vi "Panorama Generation-samples.vi"() -> ()   [LabVIEW 2023]
uses:
  <vilib>/vision/Image Controls.llb/IMAQ Image.ctl
  <vilib>/vision/Calibration.llb/Distortion Model.ctl
  <vilib>/vision/Calibration.llb/Distortion Model Types.ctl
  <vilib>/vision/EDVR.llb/IMAQ ImageToEDVR 2D SGL.vi
  <vilib>/vision/EDVR.llb/IMAQ ImageToEDVR 2D U8.vi
  <vilib>/vision/NI_Vision_Development_Module.lvlib
panel:
  in  "?":T1(tab)
  in  "?":enum32{"Processing Time  Display Tab"}(tab)
  out "SSIM Flat":dbl
  out "SSIM Original":dbl
  out "Correction":dbl
  out "Flat Fielding":dbl
  out "ROI Blending":dbl
  out "Processed FPS":dbl
  in  "Stop":bool
  out "Original Luma?":bool
  out "Left corrected, adjusted, and wrapped image":T2(plugin-control) caption="Thresholded Grid"
  out "Right corrected, adjusted, and wrapped image":T2(plugin-control) caption="Thresholded Grid"
  out "Right Sample":T2(plugin-control) caption="Thresholded Grid"
  out "Left Sample":T2(plugin-control) caption="Thresholded Grid"
  out "Panorama Image":T2(plugin-control)
  in  "?":enum32{"Tunning Control Tab"}(tab)
  in  "Right Image Name":string="right.png"
  in  "Left Image Name":string="left.png"
  in  "Wrapping Factor":i32=5
  in  "Correction Interpolation":u32(ring) items=["Zero Order", "Bi-Linear", "Quadratic", "Cubic Spline"]
  in  "Grid Path":path
  in  "Blending Method":enum16{"WA", "MBB", "WE"}(ring)
  in  "Grid Name":string="grid.png"
  in  "ROI_X":i32=10
  out "Right corrected, adjusted, and wrapped grid":T2(plugin-control) caption="Right  corrected wrapped grid"
  out "Left corrected, adjusted, and wrapped grid":T2(plugin-control) caption="Left corrected  and wrapped grid"
  out "Thresholded and filtered grid":T2(plugin-control) caption="Thresholded Grid"
  out "Grid Image":T2(plugin-control) caption="Circular Dotted Grid"
  out "ROI_L":T2(plugin-control)
  out "ROI_R":T2(plugin-control)
  out "Blended ROI":T2(plugin-control)
  out "Wrapped Y":i32
  out "Grid X":i32
  out "Grid Y":i32
  out "corrected":T2[](array[typedef])
  out "Adjusted":T2[](array[typedef])
  out "RGB Left":T2[](array[typedef])
  out "RGB Right":T2[](array[typedef])
  out "Y0":dbl
  out "X0":dbl
  out "Y1":dbl
  out "X1":dbl
  out "Y2":dbl
  out "X2":dbl
  out "Wrapped X":i32
  out "GP":T2[][](array[typedef])
  out "LP":T2[][](array[typedef])
  out "Masked RGB Right MBB":T2[](array[typedef])
  out "Masked RGB Left MBB":T2[](array[typedef])
  out "Combined Laplace":T2[][](array[typedef])
  out "Start Time":dbl
  out "Correction End Time":dbl
  out "Flat Fielding End Time":dbl
  out "Blending End Time":dbl
  out "Wrapped":T2[](array[typedef])
  out "error out":errorcluster
  out "corrected size":cluster{"X Resolution":i32, "Y Resolution":i32}
  # "This VI meticulously generates panoramic images through a carefully structured process:\n\nLens Distortion Correction: Specifically addressing Barrel Distortion to ensure precise visual accuracy.\nBrightness Variation Compensation: Achieving a seamless transition by compensating variations in brightness.\nROI Blending: Merging carefully determined Regions of Interest (ROIs) using a selected method (Weighted Average - Default, Multi-Band Blending, Wavelet Extraction).\nFinal Panorama Output: Projecting the corrected and blended elements to produce the ultimate panorama.\n\nUser Steps: Navigate to the \"Tuning Control Tab\" and follow these steps:\n\nSelect Grid Image Path: Specify the path for the grid image.\nInput Grid Image Name: Enter the grid image name as saved in the device, including its extension.\nChoose Left and Right Cameras: Indicate the cameras for the left and right images.\nCorrection Interpolation Type: Determine the interpolation type for the correction process (Zero-Order, or Bilinear).\nSet Wrapping Factor: Define the wrapping factor based on the angle between the cameras.\nROI Resolution: Specify the resolution for the Regions of Interest (ROIs).\nBlending Method: Select the preferred blending method (Weighted Average - Default, Multi-Band Blending, Wavelet Extraction).\nRun the VI."
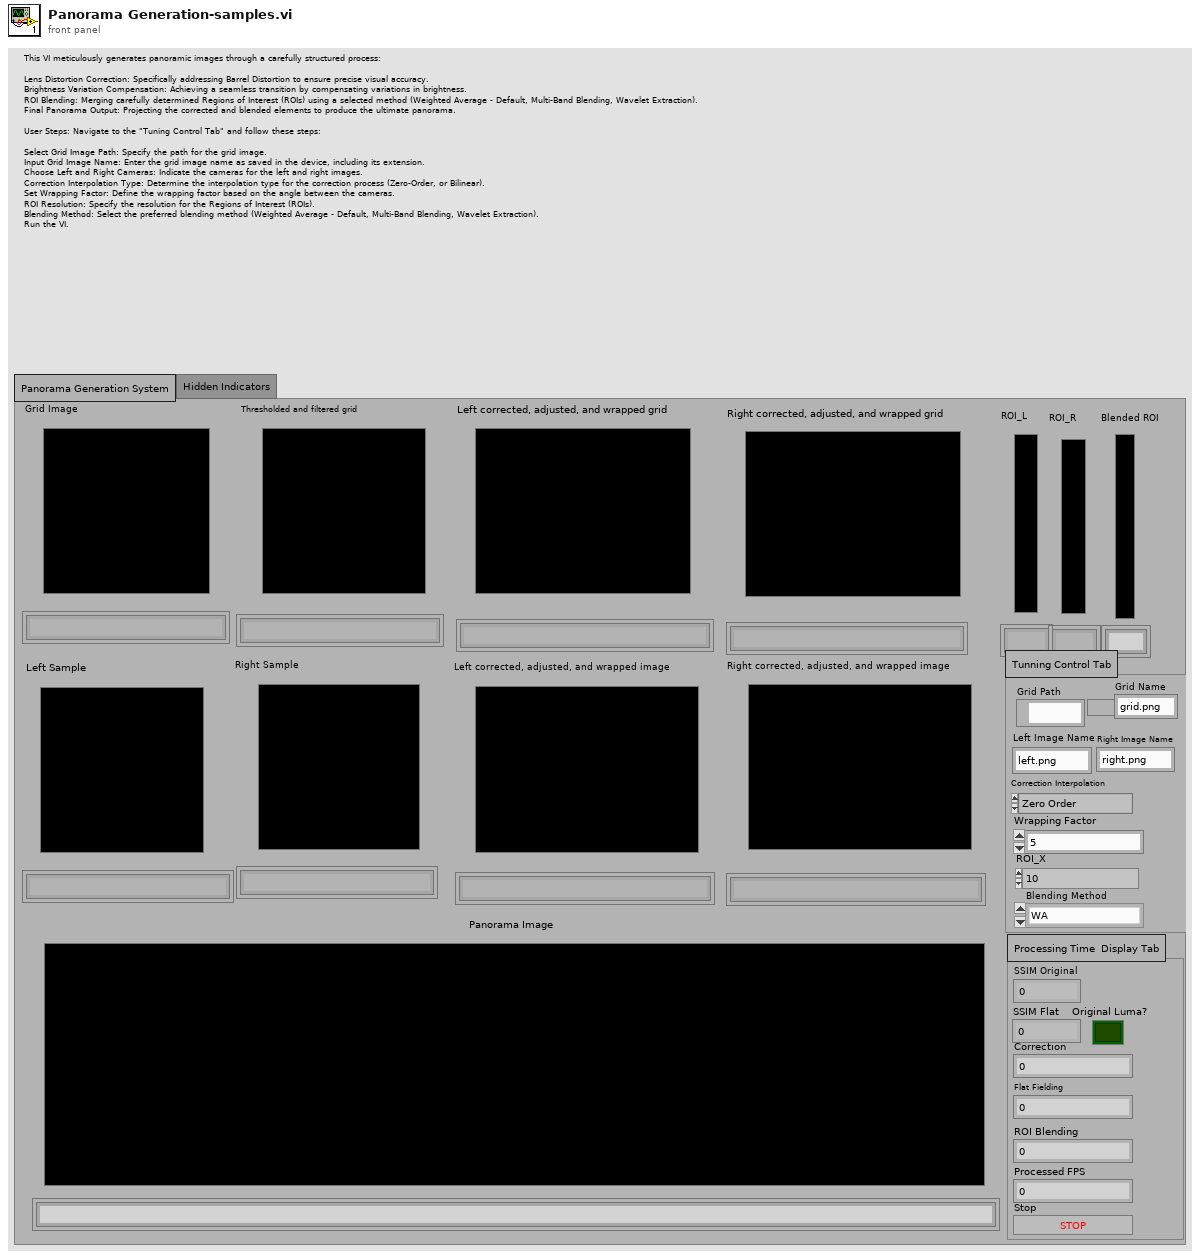
[diagram p1: front panel]
types:
  T1 = enum32{"Panorama Generation System", "Hidden Indicators"}
  T2 = typedef "IMAQ Image.ctl" = refnum<image>
  T3 = typedef "Image Unit" = enum32{"Undefined", "Angström", "Micrometer", "Millimeter", "Centimeter", "Meter", "Kilometer", "Microinch", "Inch", "Feet", "Nautical miles", "Standard miles", "Steps"}
  T4 = typedef "Particle Parameters" = i32
  T5 = cluster{"Measurement Parameter":T4, "Range Lower Value":dbl, "Range Upper Value":dbl, "Range":bool, "Measurement Type":bool}[]
  T6 = cluster{"Corrected Image Scaling":u32, "Corrected Image Learn ROI":u32, "Learn Correction Table?":bool}
  T7 = typedef "Distortion Model.ctl" = cluster{"Distortion Model":T8, "Polynomial Model Setup":cluster{"Radial Coefficient":u32, "Tangential Coefficients ":bool}}
  T8 = typedef "Distortion Model Types.ctl" = i32
  T9 = typedef "Image Type" = u32
  T10 = typedef "Calibration Reference Points.ctl" = cluster{"Pixel Coordinates":cluster{"X":dbl, "Y":dbl}[], "Real World Coordinates":cluster{"X":dbl, "Y":dbl}[], "Unit":T3, "Image Size":cluster{"X":u32, "Y":u32}}
  T11 = cluster{cluster{"element":dbl, "element":dbl}[], cluster{"element":dbl, "element":dbl}[], "Unit":T3, cluster{"X Resolution":i32, "Y Resolution":i32}}
  T12 = cluster{"Model":i32, "corrected size":cluster{"X Resolution":i32, "Y Resolution":i32}, "Polynomial Degree":i32}
  T13 = cluster{"Estimate Background?":bool, "Method":i32, "Polynomial Degree":i32, "corrected size":cluster{"X Resolution":i32, "Y Resolution":i32}, "Niblack Deviation Factor (0.2)":dbl}
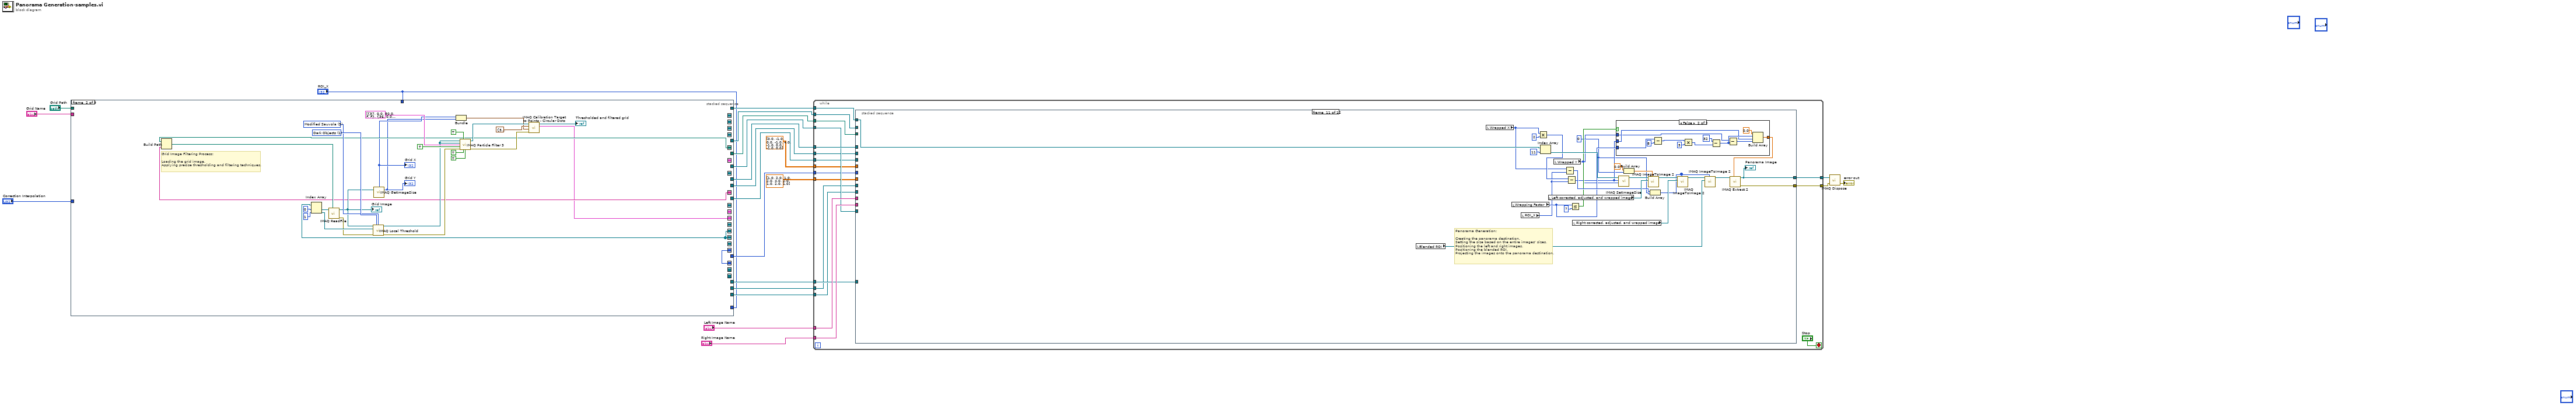
[diagram p0: block diagram]
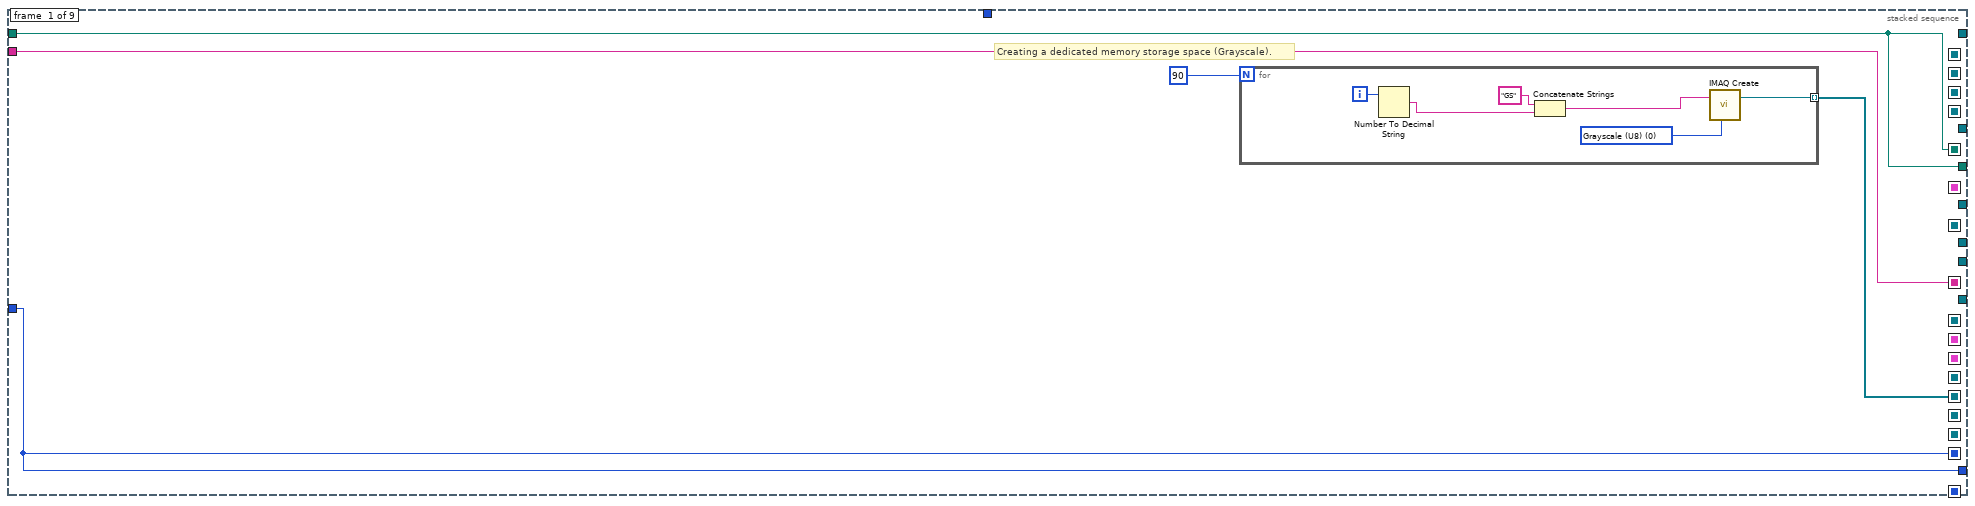
[diagram p2: hidden frame]
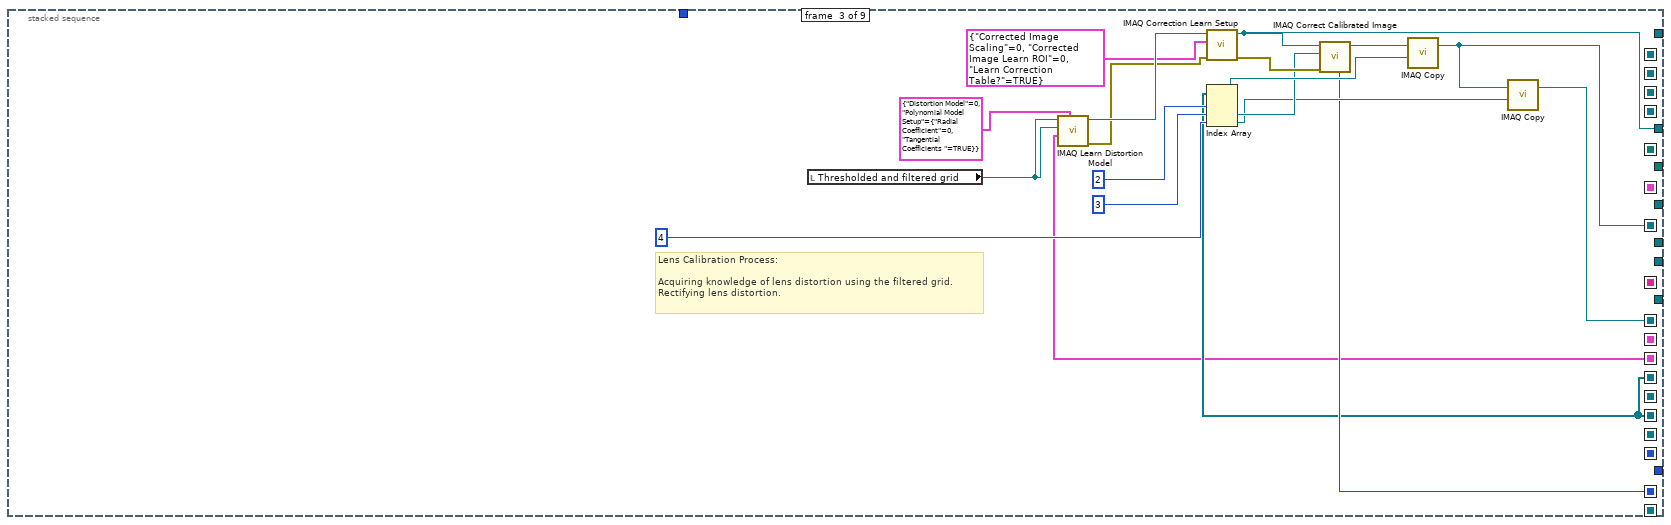
[diagram p3: hidden frame]
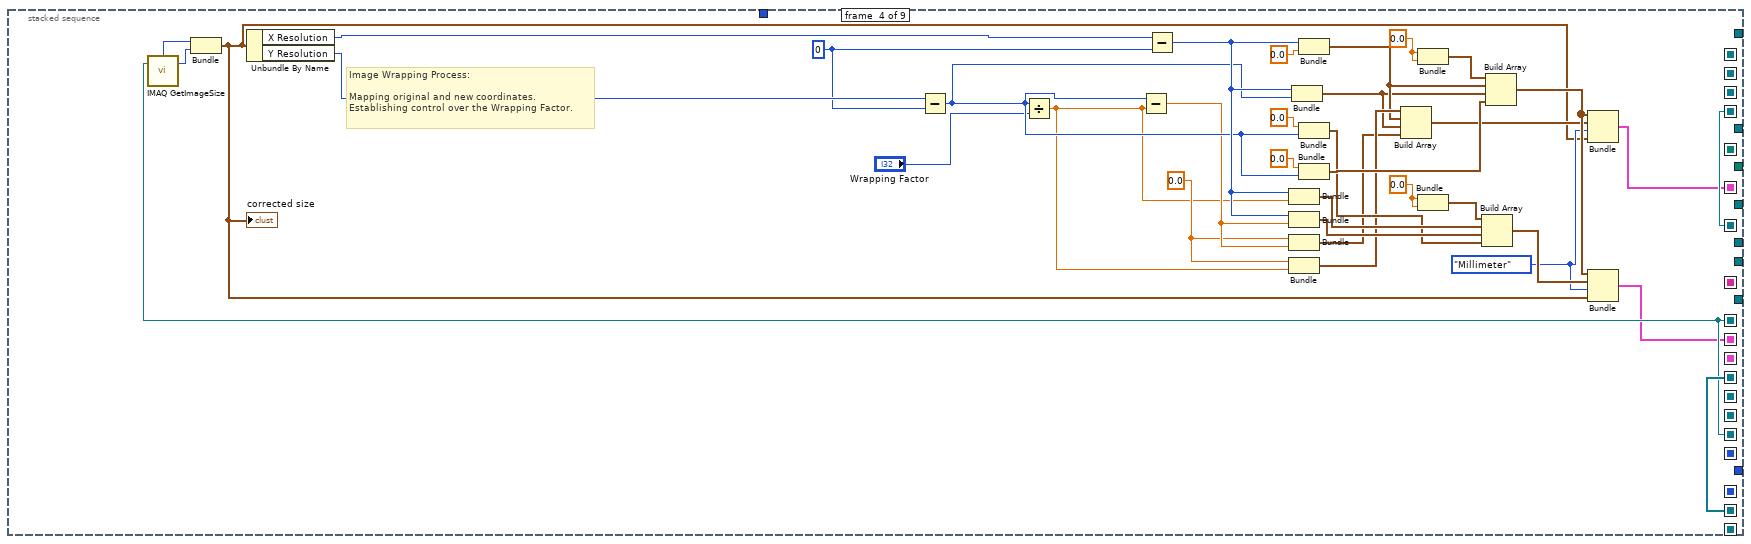
[diagram p4: hidden frame]
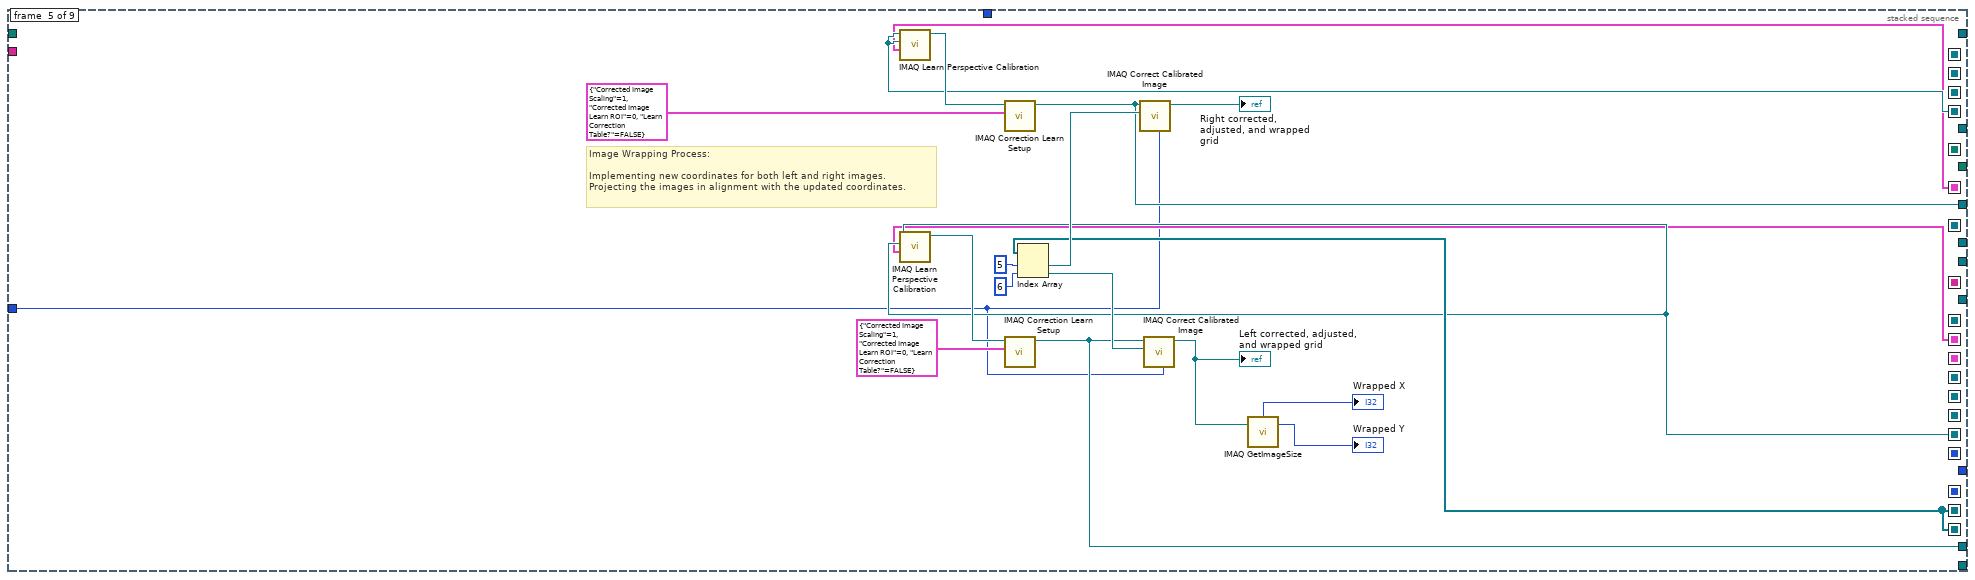
[diagram p5: hidden frame]
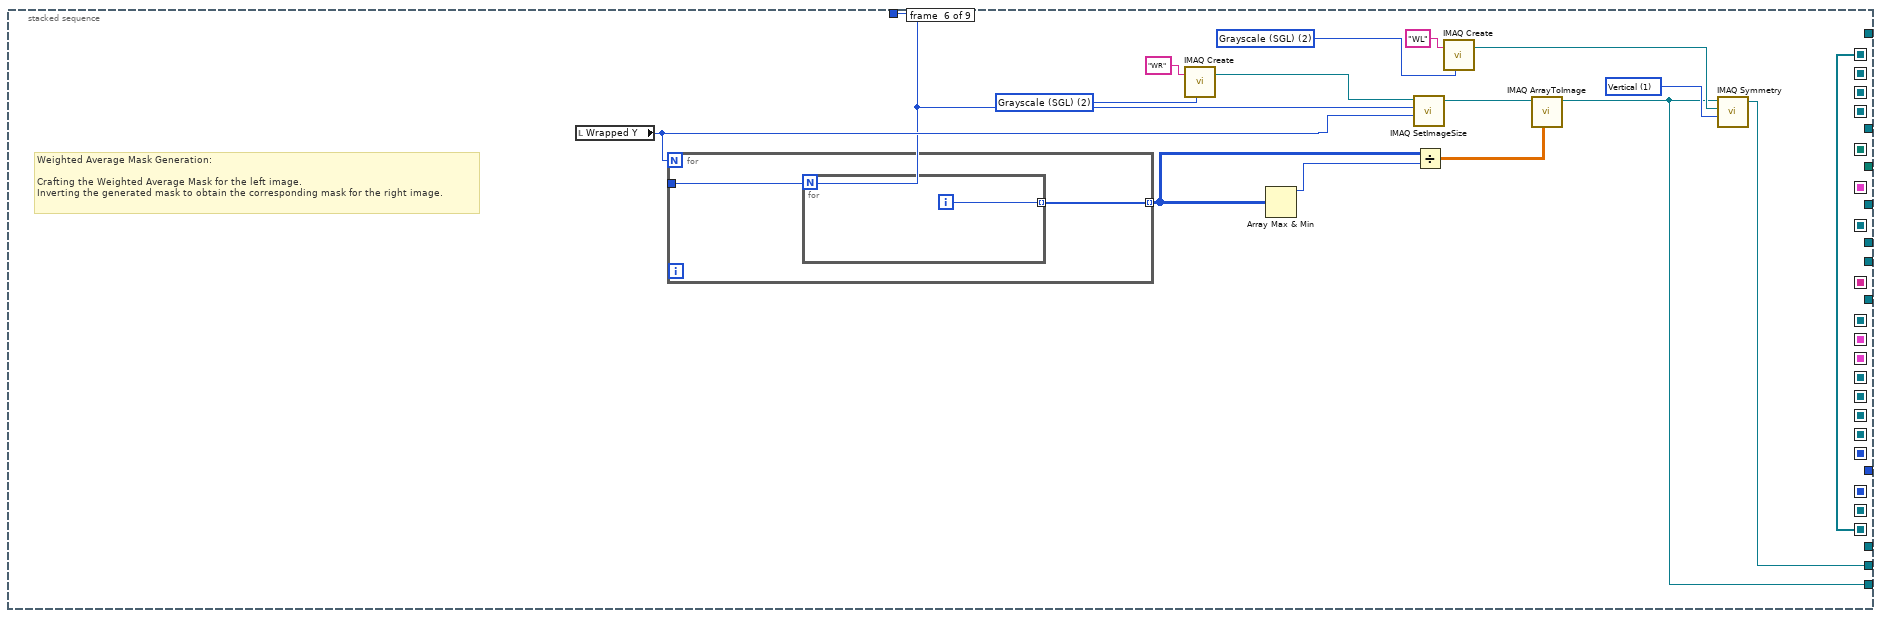
[diagram p6: hidden frame]
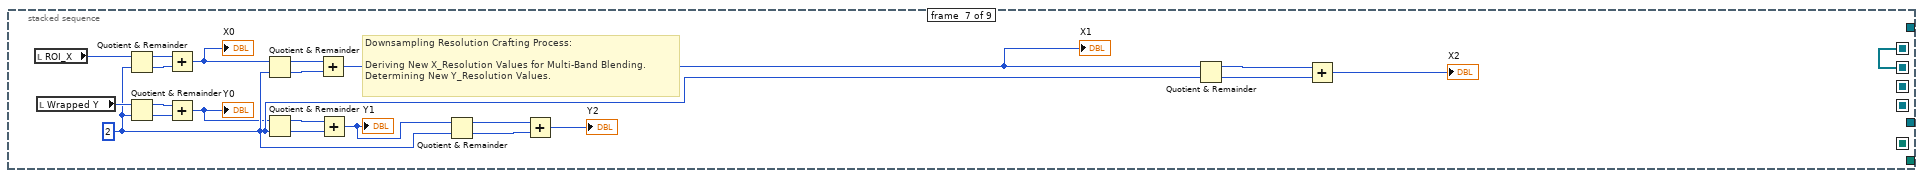
[diagram p7: hidden frame]
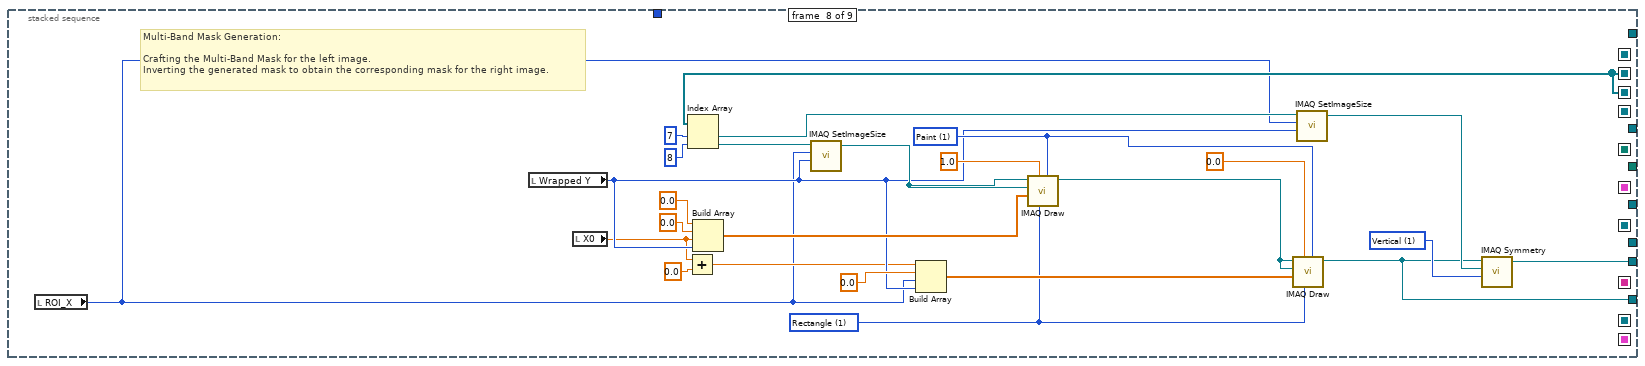
[diagram p8: hidden frame]
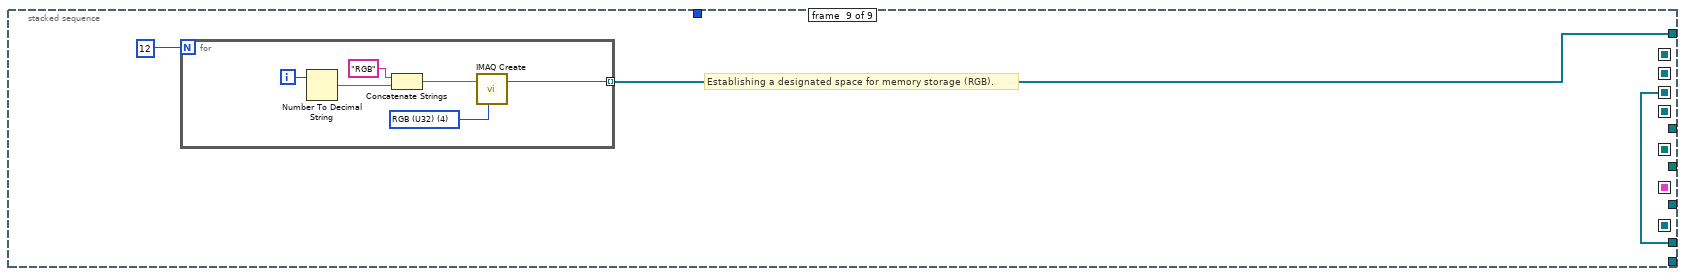
[diagram p9: hidden frame]
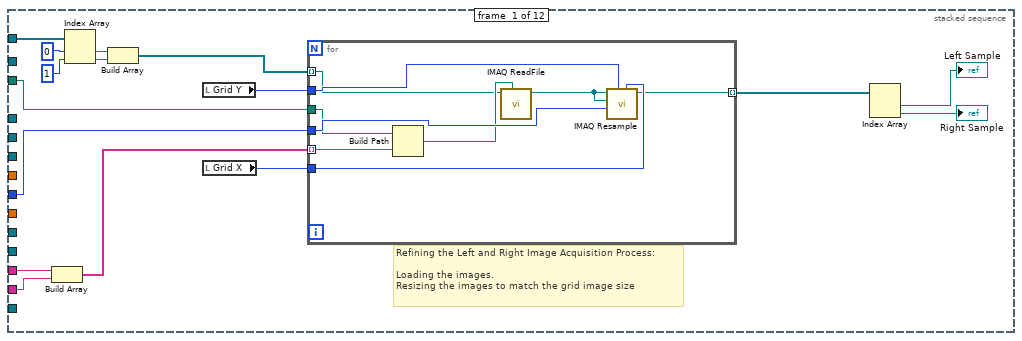
[diagram p10: hidden frame]
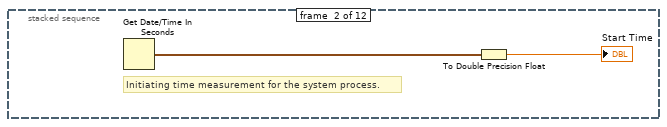
[diagram p11: hidden frame]
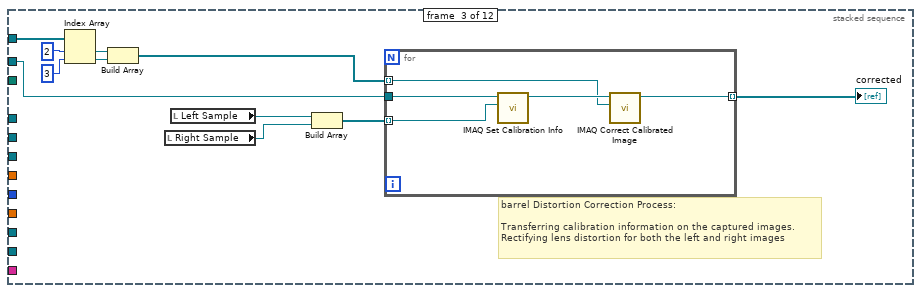
[diagram p12: hidden frame]
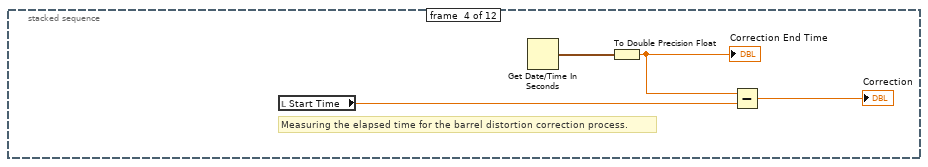
[diagram p13: hidden frame]
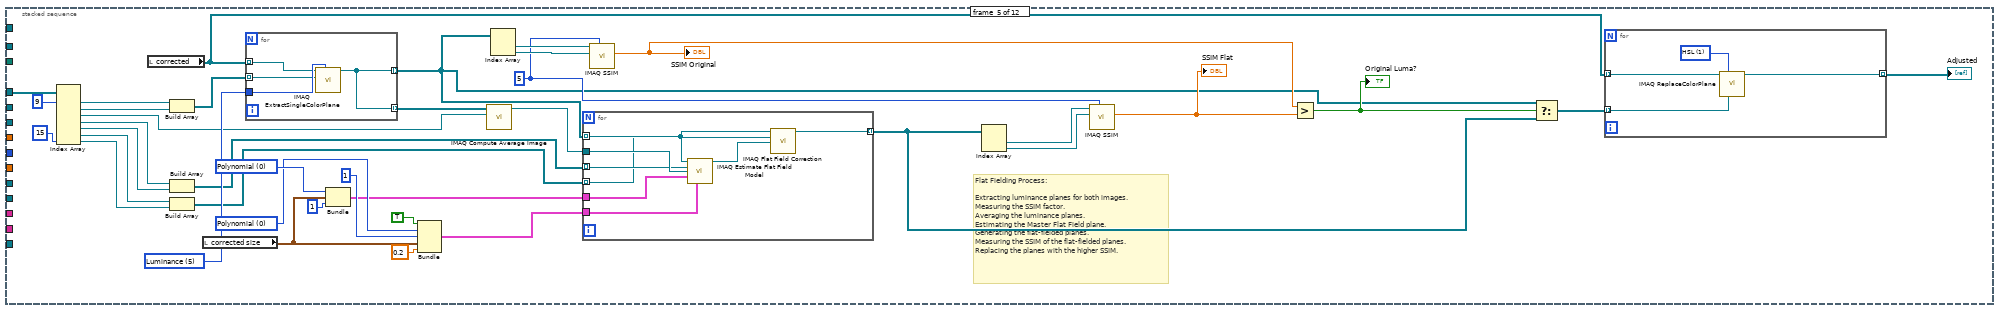
[diagram p14: hidden frame]
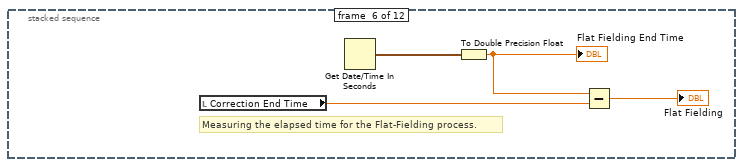
[diagram p15: hidden frame]
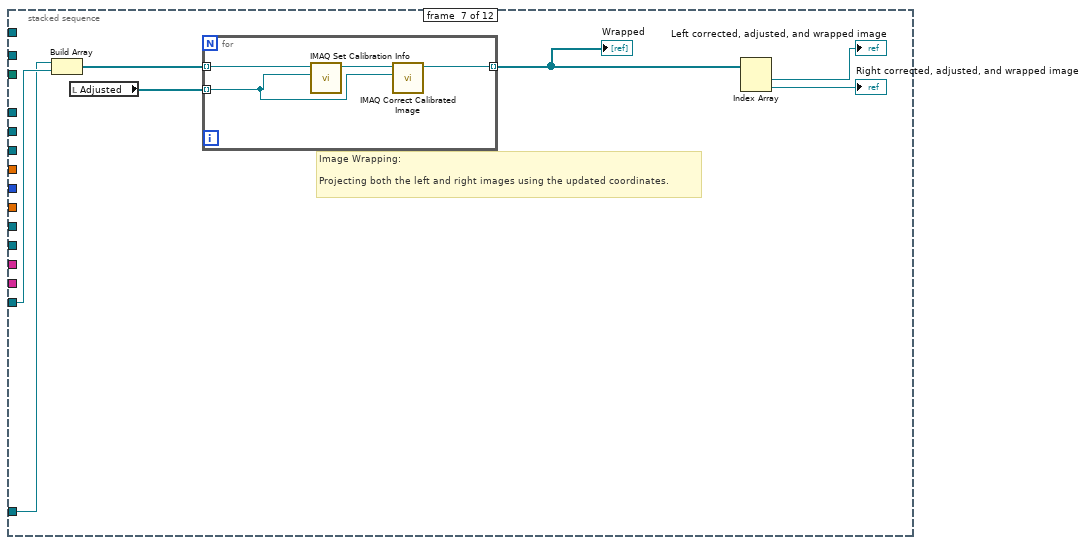
[diagram p16: hidden frame]
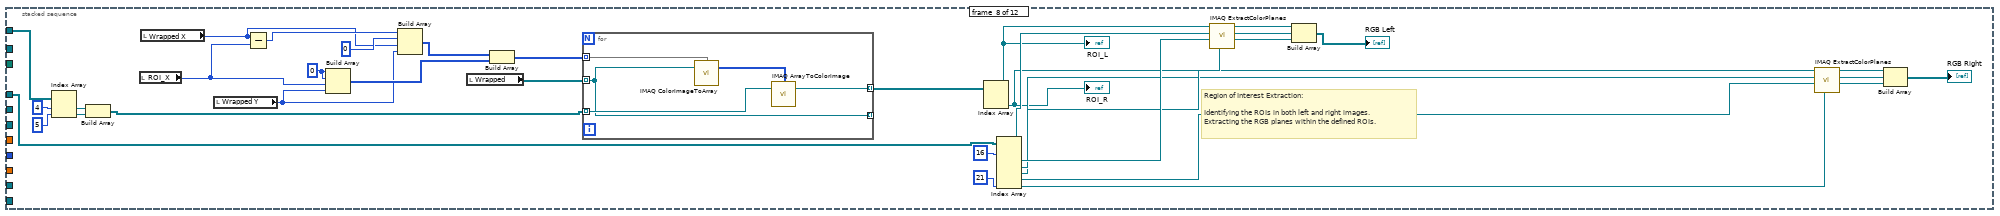
[diagram p17: hidden frame]
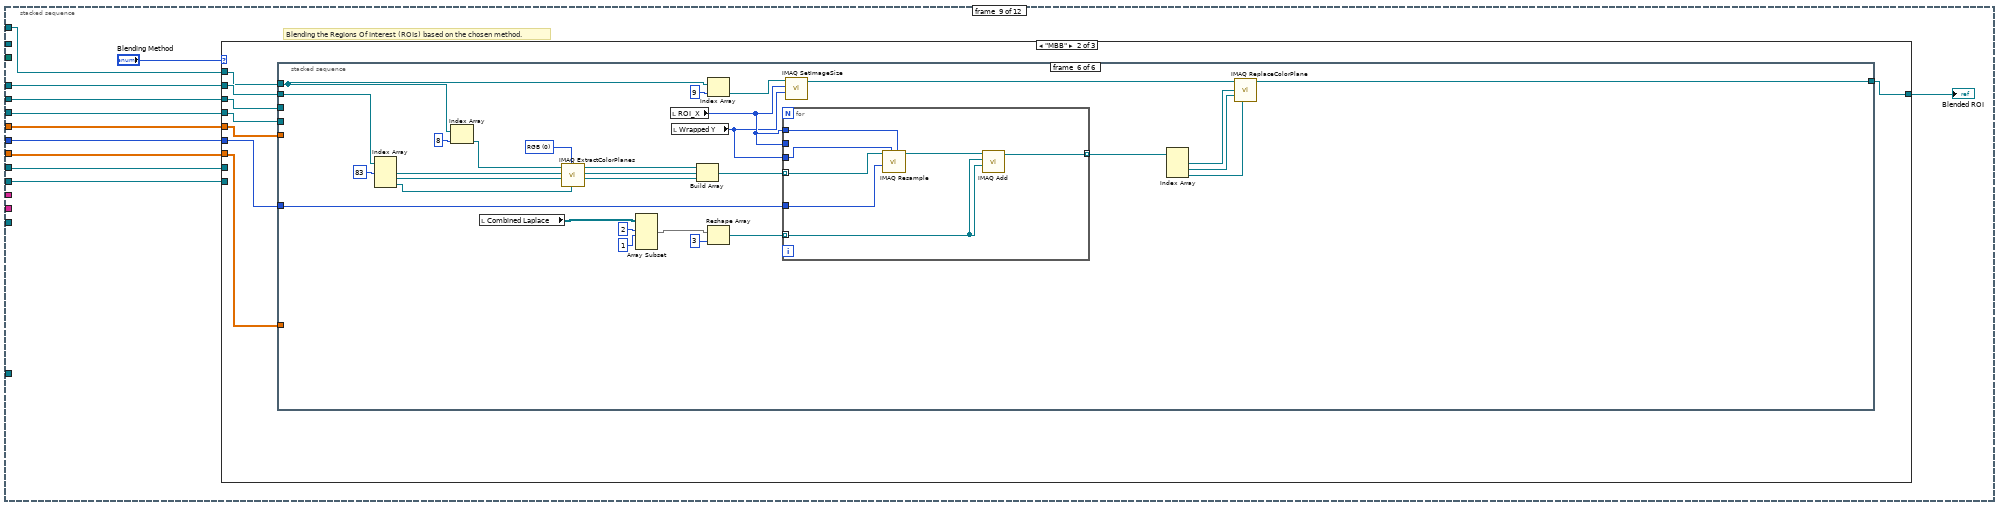
[diagram p18: hidden frame]
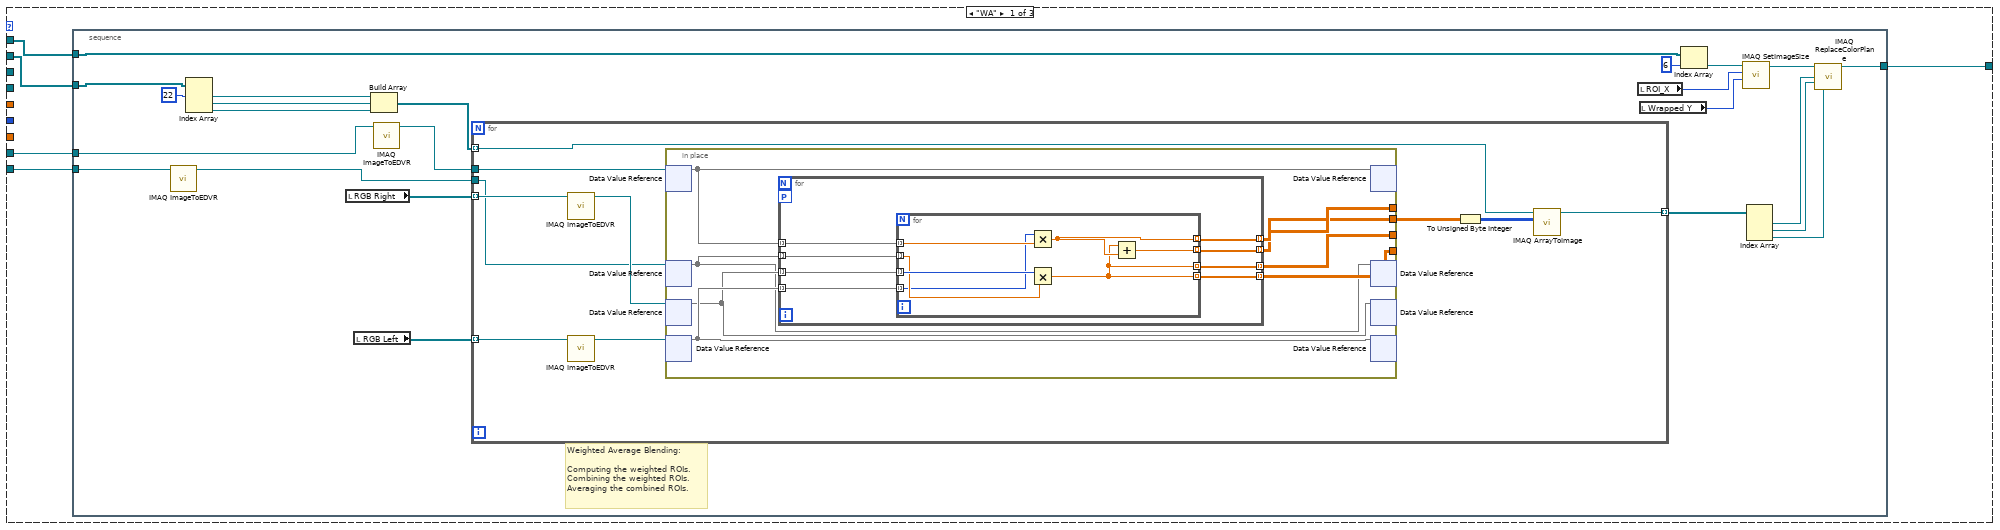
[diagram p19: hidden frame]
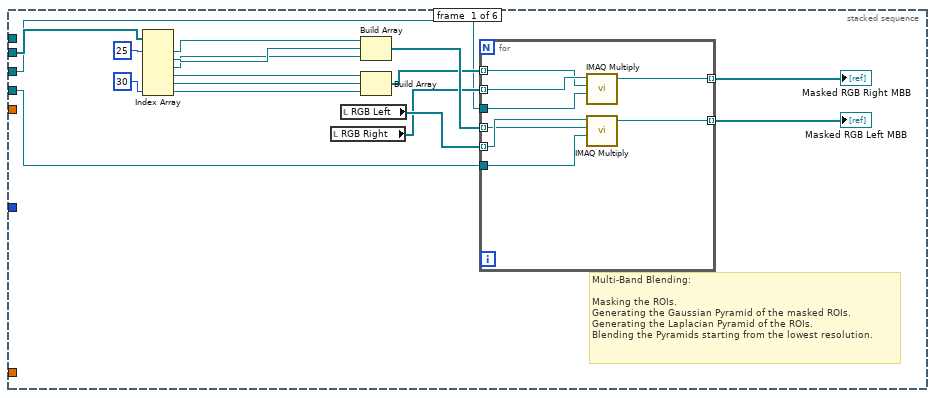
[diagram p20: hidden frame]
diagram:
  n1 = stacked-sequence {
    seq-local: [w24 _ _ _ _ _ _ _ _] -> [_ w40 _ _ _ _ _ _ _]
    seq-local: [w26 _ _ _ _ _ _ _ _] -> [_ w39 _ _ _ _ _ _ _]
    seq-local: [w23 _ _ _ _ _ _ _ _] -> [_ w38 _ _ _ _ _ _ _]
    seq-local: [w25 _ _ _ _ _ _ _ _] -> [_ w37 _ _ _ _ _ _ _]
    seq-local: [_ w38 _ _ _ _ _ _ _] -> [_ _ w67 _ _ _ _ _ _]
    seq-local: [_ w37 _ _ _ _ _ _ _] -> [_ _ w66 _ _ _ _ _ _]
    seq-local: [_ w34 _ _ _ _ _ _ _] -> [_ _ w62 _ _ _ _ _ _]
    seq-local: [_ _ w66 _ _ _ _ _ _] -> [_ _ _ w89 _ _ _ _ _]
    seq-local: [_ _ w65 _ _ _ _ _ _] -> [_ _ _ w88 _ _ _ _ _]
    seq-local: [_ _ w64 _ _ _ _ _ _] -> [_ _ _ w84 _ _ _ _ _]
    seq-local: [_ _ _ w89 _ _ _ _ _] -> [_ _ _ _ w124 _ _ _ _]
    seq-local: [_ _ _ w88 _ _ _ _ _] -> [_ _ _ _ w123 _ _ _ _]
    seq-local: [_ _ _ w84 _ _ _ _ _] -> [_ _ _ _ w122 _ _ _ _]
    seq-local: [_ _ _ w83 _ _ _ _ _] -> [_ _ _ _ w121 _ _ _ _]
    seq-local: [_ _ _ w82 _ _ _ _ _] -> [_ _ _ _ w120 _ _ _ _]
    seq-local: [_ _ _ _ w124 _ _ _ _] -> [_ _ _ _ _ w140 _ _ _]
    seq-local: [_ _ _ _ _ w140 _ _ _] -> [_ _ _ _ _ _ w156 _ _]
    seq-local: [_ _ _ _ _ _ w156 _ _] -> [_ _ _ _ _ _ _ w181 _]
    seq-local: [_ _ _ _ _ _ _ w181 _] -> [_ _ _ _ _ _ _ _ w205]
    tunnel: "Grid Path" -> [w24 _ _ _ _ _ _ _ _]
    tunnel: "Grid Name" -> [w26 _ _ _ _ _ _ _ _]
    tunnel: "Correction Interpolation" -> [w23 _ _ _ w117 _ _ _ _]
    tunnel: [_ _ w63 _ _ _ _ _ _] -> w10
    tunnel: [_ _ _ _ w119 _ _ _ _] -> w8
    tunnel: [_ _ _ _ w118 _ _ _ _] -> w9
    tunnel: [_ _ _ _ _ _ _ w180 _] -> w6
    tunnel: [_ _ _ _ _ _ _ w179 _] -> w7
    tunnel: [_ _ _ _ _ _ _ _ w205] -> w12
    tunnel: [_ _ _ _ _ _ _ _ w203] -> w11
    tunnel: [_ _ _ _ _ w139 _ _ _] -> w5
    tunnel: [_ _ _ _ _ w138 _ _ _] -> w4
    tunnel: [w24 _ _ _ _ _ _ _ _] -> w3
    tunnel: [w23 _ _ _ _ _ _ _ _] -> w2
    tunnel: "ROI_X" -> [_ _ _ _ _ _ _ _ _]
    tunnel: "ROI_X" -> [_ _ _ _ _ w137 _ _ _]
    tunnel: [_ _ _ _ _ w137 _ _ _] -> _
    frame #0 {
      # "Creating a dedicated memory storage space (Grayscale)."
      n2 = for {
        N: 90 -> [_]
        tunnel: [w28] -> w25 mode=indexing
        i -> [w29]
        w30 = T9 0 items=["Grayscale (U8)", "Grayscale (I16)", "Grayscale (SGL)", "Complex (CSG)", "RGB (U32)", "HSL (U32)", "RGB (U64)", "Grayscale (U16)"] ("Image Type")
        n3 = Number To Decimal String(number=w29) -> (decimal integer string=w33:string)  [unwired: 1 out]
        n4 = Concatenate Strings("GS" ("string"), w33) -> (w32:string)
        n5 = call "IMAQ Create"("Image Name"=w32, "Image Type"=w30) -> ("New Image"=w28:T2)  [unwired: 2 in, 2 out]
      }
    }
    frame #1 {
      w53 = u32 3 items=["Niblack", "Background Correction", "Sauvola", "Modified Sauvola"] ("Method (Niblack)")
      w54 = u32 1 items=["Bright Objects", "Dark Objects"] ("Look For (Bright Objects)")
      # "Grid Image Filtering Process:\n\nLoading the grid image.\nApplying precise thresholding and filtering techniques."
      n6 = Build Path(base path=w40, name or relative path=w39) -> (appended path=w61:path)
      n7 = Index Array(array=w37, index #1=0 ("index"), index #2=1 ("index")) -> (element #1=w51:T2, element #2=w50:T2)
      n8 = call "IMAQ ReadFile"("File Path"=w61, "Image"=w51) -> ("error out"=w41:errorcluster, "Image Out"=w42:T2)  [unwired: 3 in, 5 out]
      "Grid Image" <- w42
      n9 = call "IMAQ Local Threshold"("Image Src"=w42, "Look For (Bright Objects)"=w54, "Method (Niblack)"=w53, "Image Dst"=w50, "error in (no error)"=w41) -> ("Image Dst Out"=w48:T2, "error out"=w60:errorcluster)  [unwired: 9 in]
      n10 = call "IMAQ GetImageSize"("Image"=w42) -> ("Y Resolution"=w35:i32, "X Resolution"=w36:i32)  [unwired: 3 in, 1 out]
      "Grid X" <- w36
      "Grid Y" <- w35
      n11 = Bundle("X Resolution"=w36, "Y Resolution"=w35) -> (w43:cluster{"X Resolution":i32, "Y Resolution":i32})  [unwired: 1 in]
      n12 = call "IMAQ Particle Filter 3"("Image Src"=w48, "Connectivity 4/8 (8)"=TRUE, "Image Dst"=w48, "Selection Values"=T5 [{"Measurement Parameter"=37, "Range Lower Value"=0.0, "Range Upper Value"=50.0, "Range"=FALSE, "Measurement Type"=FALSE}, {"Measurement Parameter"=36, "Range Lower Value"=0.0, "Range Upper Value"=0.0, "Range"=FALSE, "Measurement Type"=FALSE}], "Keep/Remove Particles (F)"=TRUE, "error in (no error)"=w60, "Reject Border? (F)"=TRUE, "Fill Holes? (F)"=TRUE) -> ("Image Dst Out"=w44:T2, "error out"=w45:errorcluster)  [unwired: 1 in, 5 out]
      n13 = call "IMAQ Calibration Target to Points - Circular Dots"("error in (no error)"=w45, "Grid Size"=w43, "Grid Descriptor"=cluster{"X Step":sgl, "Y Step":sgl, "Unit":T3} {"X Step"=3.6, "Y Step"=3.6, "Unit"=enum."Millimeter"}, "Target Image"=w44) -> ("Reference Points"=w34:T10, "Target Image (dup)"=→"Thresholded and filtered grid":T2)  [unwired: 5 in, 1 out]
    }
    frame #2 {
      # "Lens Calibration Process:\n\nAcquiring knowledge of lens distortion using the filtered grid.\nRectifying lens distortion."
      n14 = local read "Thresholded and filtered grid"() -> (w71:T2)
      n15 = call "IMAQ Learn Distortion Model"("Distortion Model Setup"=T7 {"Distortion Model"=0, "Polynomial Model Setup"={"Radial Coefficient"=0, "Tangential Coefficients "=TRUE}}, "Reference Points"=w62, "Image"=w71, "Calibration Template Image"=w71) -> ("error out"=w78:errorcluster, "Calibration Template Image Out"=w79:T2)  [unwired: 6 in]
      n16 = call "IMAQ Correction Learn Setup"("error in (no error)"=w78, "Correction Learn Setup"=T6 {"Corrected Image Scaling"=0, "Corrected Image Learn ROI"=0, "Learn Correction Table?"=TRUE}, "Calibration Template Image"=w79) -> ("error out"=w77:errorcluster, "Calibration Template Image Out"=w63:T2)  [unwired: 7 in]
      n17 = Index Array(array=w66, index #1=2 ("index"), index #2=3 ("index"), index #3=4 ("index")) -> (element #1=w72:T2, element #2=w70:T2, element #3=w69:T2)
      n18 = call "IMAQ Correct Calibrated Image"("Interpolation Type"=w67, "error in (no error)"=w77, "Image Dst"=w70, "Image Src"=w63) -> ("Corrected Image"=w80:T2)  [unwired: 6 in, 1 out]
      n19 = call "IMAQ Copy"("Image Dst"=w72, "Image Src"=w80) -> ("Image Dst Out"=w65:T2)  [unwired: 4 in, 1 out]
      n20 = call "IMAQ Copy"("Image Dst"=w69, "Image Src"=w65) -> ("Image Dst Out"=w64:T2)  [unwired: 4 in, 1 out]
    }
    frame #3 {
      w98 = 0.0 ("element")
      w96 = 0 ("y")
      w94 = 0.0 ("element")
      w91 = 0.0 ("element")
      w97 = Image_Unit."Millimeter" ("Unit")
      # "Image Wrapping Process:\n\nMapping original and new coordinates.\nEstablishing control over the Wrapping Factor."
      n21 = call "IMAQ GetImageSize"("Image"=w84) -> ("Y Resolution"=w87:i32, "X Resolution"=w86:i32)  [unwired: 3 in, 1 out]
      n22 = Bundle("X Resolution"=w86, "Y Resolution"=w87) -> (w85:cluster{"X Resolution":i32, "Y Resolution":i32})  [unwired: 1 in]
      "corrected size" <- w85
      n23 = Unbundle By Name(w85) -> ("X Resolution"=w109:i32, "Y Resolution"=w108:i32)
      n24 = Subtract(x=w108, y=w96) -> (x-y=w105:i32)
      n25 = Divide(x=w105, y="Wrapping Factor") -> (x/y=w90:dbl)
      n26 = Subtract(x=w105, y=w90) -> (x-y=w101:dbl)
      n27 = Subtract(x=w109, y=w96) -> (x-y=w106:i32)
      n28 = Bundle(w106, w90) -> (w113:cluster{i32, dbl})  [unwired: 1 in]
      n29 = Bundle(w106, w101) -> (w112:cluster{i32, dbl})  [unwired: 1 in]
      n30 = Bundle("element"=w98, w101) -> (w100:cluster{"element":dbl, dbl})  [unwired: 1 in]
      n31 = Bundle("element"=w98, w90) -> (w104:cluster{"element":dbl, dbl})  [unwired: 1 in]
      n32 = Bundle(w106, w105) -> (w102:cluster{i32, i32})  [unwired: 1 in]
      n33 = Bundle(w106, "element"=0.0) -> (w103:cluster{i32, "element":dbl})  [unwired: 1 in]
      n34 = Bundle("element"=0.0, w105) -> (w111:cluster{"element":dbl, i32})  [unwired: 1 in]
      n35 = Bundle("element"=0.0, w105) -> (w115:cluster{"element":dbl, i32})  [unwired: 1 in]
      n36 = Build Array(w104, w103, w102, w100) -> (w99:cluster{"element":dbl, "element":dbl}[])
      n37 = Bundle("element"=w91, "element"=w91) -> (w116:cluster{"element":dbl, "element":dbl})  [unwired: 1 in]
      n38 = Bundle("element"=w94, "element"=w94) -> (w114:cluster{"element":dbl, "element":dbl})  [unwired: 1 in]
      n39 = Build Array(w114, w113, w112, w111) -> (w110:cluster{"element":dbl, "element":dbl}[])
      n40 = Build Array(w116, w103, w102, w115) -> (w107:cluster{"element":dbl, "element":dbl}[])
      n41 = Bundle(w107, w99, "Unit"=w97, w85) -> (w83:T11)  [unwired: 1 in]
      n42 = Bundle(w107, w110, "Unit"=w97, w85) -> (w82:T11)  [unwired: 1 in]
    }
    frame #4 {
      # "Image Wrapping Process:\n\nImplementing new coordinates for both left and right images.\nProjecting the images in alignment with the updated coordinates."
      n43 = call "IMAQ Learn Perspective Calibration"("Reference Points"=w121, "Image"=w123, "Calibration Template Image"=w123) -> ("Calibration Template Image Out"=w134:T2)  [unwired: 7 in, 1 out]
      n44 = call "IMAQ Learn Perspective Calibration"("Reference Points"=w120, "Image"=w122, "Calibration Template Image"=w122) -> ("Calibration Template Image Out"=w136:T2)  [unwired: 7 in, 1 out]
      n45 = call "IMAQ Correction Learn Setup"("Correction Learn Setup"=T6 {"Corrected Image Scaling"=1, "Corrected Image Learn ROI"=0, "Learn Correction Table?"=FALSE}, "Calibration Template Image"=w134) -> ("Calibration Template Image Out"=w119:T2)  [unwired: 8 in, 1 out]
      n46 = call "IMAQ Correction Learn Setup"("Correction Learn Setup"=T6 {"Corrected Image Scaling"=1, "Corrected Image Learn ROI"=0, "Learn Correction Table?"=FALSE}, "Calibration Template Image"=w136) -> ("Calibration Template Image Out"=w118:T2)  [unwired: 8 in, 1 out]
      n47 = Index Array(array=w124, index #1=5 ("index"), index #2=6 ("index")) -> (element #1=w129:T2, element #2=w128:T2)
      n48 = call "IMAQ Correct Calibrated Image"("Interpolation Type"=w117, "Image Dst"=w129, "Image Src"=w119) -> ("Corrected Image"=→"Right corrected, adjusted, and wrapped grid":T2)  [unwired: 7 in, 1 out]
      n49 = call "IMAQ Correct Calibrated Image"("Interpolation Type"=w117, "Image Dst"=w128, "Image Src"=w118) -> ("Corrected Image"=w125:T2)  [unwired: 7 in, 1 out]
      "Left corrected, adjusted, and wrapped grid" <- w125
      n50 = call "IMAQ GetImageSize"("Image"=w125) -> ("Y Resolution"=→"Wrapped Y":i32, "X Resolution"=→"Wrapped X":i32)  [unwired: 3 in, 1 out]
    }
    frame #5 {
      w145 = u32 1 items=["Horizontal", "Vertical", "Central", "1st Diagonal", "2nd Diagonal"] ("Type of Symmetry")
      w146 = T9 2 items=["Grayscale (U8)", "Grayscale (I16)", "Grayscale (SGL)", "Complex (CSG)", "RGB (U32)", "HSL (U32)", "RGB (U64)", "Grayscale (U16)"] ("Image Type")
      w149 = T9 2 items=["Grayscale (U8)", "Grayscale (I16)", "Grayscale (SGL)", "Complex (CSG)", "RGB (U32)", "HSL (U32)", "RGB (U64)", "Grayscale (U16)"] ("Image Type")
      # "Weighted Average Mask Generation:\n\nCrafting the Weighted Average Mask for the left image.\nInverting the generated mask to obtain the corresponding mask for the right image."
      n51 = local read "Wrapped Y"() -> (w144:i32)
      n52 = for {
        N: w144 -> [_]
        tunnel: [w154] -> w142 mode=indexing
        tunnel: w137 -> [w153]
        n53 = for {
          N: w153 -> [_]
          tunnel: [w155] -> w154 mode=indexing
          i -> [w155]
        }
      }
      n54 = call "IMAQ Create"("Image Name"="WR", "Image Type"=w149) -> ("New Image"=w151:T2)  [unwired: 2 in, 2 out]
      n55 = Array Max & Min(array=w142) -> (max value=w141:i32)  [unwired: 3 out]
      n56 = call "IMAQ SetImageSize"("Y Resolution"=w144, "X Resolution"=w137, "Image"=w151) -> ("Image Out"=w150:T2)  [unwired: 2 in, 1 out]
      n57 = Divide(x=w142, y=w141) -> (x/y=w143:dbl[][])
      n58 = call "IMAQ Create"("Image Name"="WL", "Image Type"=w146) -> ("New Image"=w148:T2)  [unwired: 2 in, 2 out]
      n59 = call "IMAQ ArrayToImage"("Image Pixels (Float)"=w143, "Image"=w150) -> ("Image Out"=w138:T2)  [unwired: 8 in, 1 out]
      n60 = call "IMAQ Symmetry"("Type of Symmetry"=w145, "Image Dst"=w148, "Image Src"=w138) -> ("Image Dst Out"=w139:T2)  [unwired: 2 in, 1 out]
    }
    frame #6 {
      w163 = 2 ("y")
      # "Downsampling Resolution Crafting Process:\n\nDeriving New X_Resolution Values for Multi-Band Blending.\nDetermining New Y_Resolution Values."
      n61 = local read "ROI_X"() -> (w177:i32)
      n62 = local read "Wrapped Y"() -> (w176:i32)
      n63 = Quotient & Remainder(x=w177, y=w163) -> (x-y*floor(x/y)=w175:i32, floor(x/y)=w174:i32)
      n64 = Quotient & Remainder(x=w176, y=w163) -> (x-y*floor(x/y)=w173:i32, floor(x/y)=w172:i32)
      n65 = Add(x=w175, y=w174) -> (x+y=w157:i32)
      "X0" <- w157
      n66 = Add(x=w173, y=w172) -> (x+y=w160:i32)
      "Y0" <- w160
      n67 = Quotient & Remainder(x=w157, y=w163) -> (x-y*floor(x/y)=w169:i32, floor(x/y)=w168:i32)
      n68 = Quotient & Remainder(x=w160, y=w163) -> (x-y*floor(x/y)=w171:i32, floor(x/y)=w170:i32)
      n69 = Add(x=w169, y=w168) -> (x+y=w158:i32)
      "X1" <- w158
      n70 = Add(x=w171, y=w170) -> (x+y=w161:i32)
      "Y1" <- w161
      n71 = Quotient & Remainder(x=w161, y=w163) -> (x-y*floor(x/y)=w167:i32, floor(x/y)=w166:i32)
      n72 = Add(x=w167, y=w166) -> (x+y=→"Y2":i32)
      n73 = Quotient & Remainder(x=w158, y=w163) -> (x-y*floor(x/y)=w165:i32, floor(x/y)=w164:i32)
      n74 = Add(x=w165, y=w164) -> (x+y=→"X2":i32)
    }
    frame #7 {
      w185 = u32 1 items=["Horizontal", "Vertical", "Central", "1st Diagonal", "2nd Diagonal"] ("Type of Symmetry")
      w189 = u16 1 items=["Line", "Rectangle", "Oval"] ("Shape to draw")
      w196 = u16 1 items=["Frame", "Paint", "Invert Frame", "Invert Paint"] ("Draw Mode")
      # "Multi-Band Mask Generation:\n\nCrafting the Multi-Band Mask for the left image.\nInverting the generated mask to obtain the corresponding mask for the right image."
      n75 = local read "ROI_X"() -> (w178:i32)
      n76 = local read "Wrapped Y"() -> (w186:i32)
      n77 = local read "X0"() -> (w182:dbl)
      n78 = Add(x=w182, y=0.0) -> (x+y=w183:dbl)
      n79 = Index Array(array=w181, index #1=7 ("index"), index #2=8 ("index")) -> (element #1=w187:T2, element #2=w199:T2)
      n80 = Build Array(0.0 ("element"), 0.0 ("element"), w182, w186) -> (w191:dbl[])
      n81 = call "IMAQ SetImageSize"("Y Resolution"=w186, "X Resolution"=w178, "Image"=w199) -> ("Image Out"=w198:T2)  [unwired: 2 in, 1 out]
      n82 = Build Array(w183, 0.0 ("element"), w178, w186) -> (w194:dbl[])
      n83 = call "IMAQ Draw"("Draw Mode"=w196, "Shape to draw"=w189, "Pixel Color"=sgl 1.0, "Coordinates"=w191, "Image Dst"=w198, "Image Src"=w198) -> ("Image Dst Out"=w195:T2)  [unwired: 4 in, 1 out]
      n84 = call "IMAQ Draw"("Draw Mode"=w196, "Shape to draw"=w189, "Pixel Color"=sgl 0.0, "Coordinates"=w194, "Image Dst"=w195, "Image Src"=w195) -> ("Image Dst Out"=w180:T2)  [unwired: 4 in, 1 out]
      n85 = call "IMAQ SetImageSize"("Y Resolution"=w186, "X Resolution"=w178, "Image"=w187) -> ("Image Out"=w188:T2)  [unwired: 2 in, 1 out]
      n86 = call "IMAQ Symmetry"("Type of Symmetry"=w185, "Image Dst"=w188, "Image Src"=w180) -> ("Image Dst Out"=w179:T2)  [unwired: 2 in, 1 out]
    }
    frame #8 {
      # "Establishing a designated space for memory storage (RGB)."
      n87 = for {
        N: 12 -> [_]
        tunnel: [w207] -> w203 mode=indexing
        i -> [w206]
        w208 = T9 4 items=["Grayscale (U8)", "Grayscale (I16)", "Grayscale (SGL)", "Complex (CSG)", "RGB (U32)", "HSL (U32)", "RGB (U64)", "Grayscale (U16)"] ("Image Type")
        n88 = Number To Decimal String(number=w206) -> (decimal integer string=w211:string)  [unwired: 1 out]
        n89 = Concatenate Strings("RGB" ("string"), w211) -> (w210:string)
        n90 = call "IMAQ Create"("Image Name"=w210, "Image Type"=w208) -> ("New Image"=w207:T2)  [unwired: 2 in, 2 out]
      }
    }
  }
  n91 = while {
    tunnel: w3 -> [w228]
    tunnel: "Right Image Name" -> [w227]
    tunnel: "Left Image Name" -> [w226]
    tunnel: w11 -> [w225]
    tunnel: w10 -> [w224]
    tunnel: w12 -> [w223]
    tunnel: w8 -> [w222]
    tunnel: w9 -> [w221]
    tunnel: w7 -> [w220]
    tunnel: w6 -> [w219]
    tunnel: w5 -> [w218]
    tunnel: w4 -> [w217]
    tunnel: w2 -> [w216]
    tunnel: sgl[][] [[1.0, 2.0, 1.0], [2.0, 4.0, 2.0], [1.0, 2.0, 1.0]] ("Gaussian Kernel") -> [w215]
    tunnel: sgl[][] [[0.0, -1.0, 0.0], [-1.0, 4.0, -1.0], [0.0, -1.0, 0.0]] ("Laplace Kernel 2") -> [w214]
    tunnel: [w213] -> w16
    tunnel: [w212] -> w15
    stop <- "Stop" stop-if-true
    n92 = stacked-sequence {
      tunnel: w228 -> [w234 _ _ _ _ _ _ _ _ _ _ _]
      tunnel: w227 -> [w233 _ _ _ _ _ _ _ _ _ _ _]
      tunnel: w226 -> [w232 _ _ _ _ _ _ _ _ _ _ _]
      tunnel: w225 -> [w231 _ w258 _ _ _ _ w351 w395 _ w786 _]
      tunnel: w224 -> [_ _ w257 _ _ _ _ _ _ _ _ _]
      tunnel: w223 -> [_ _ _ _ w292 _ _ w350 w396 _ _ _]
      tunnel: w222 -> [_ _ _ _ _ _ w336 _ _ _ _ _]
      tunnel: w221 -> [_ _ _ _ _ _ w335 _ _ _ _ _]
      tunnel: w220 -> [_ _ _ _ _ _ _ _ w388 _ _ _]
      tunnel: w219 -> [_ _ _ _ _ _ _ _ w387 _ _ _]
      tunnel: w218 -> [_ _ _ _ _ _ _ _ w394 _ _ _]
      tunnel: w217 -> [_ _ _ _ _ _ _ _ w393 _ _ _]
      tunnel: w216 -> [w230 _ _ _ _ _ _ _ w392 _ _ _]
      tunnel: w215 -> [_ _ _ _ _ _ _ _ w391 _ _ _]
      tunnel: w214 -> [_ _ _ _ _ _ _ _ w390 _ _ _]
      tunnel: [_ _ _ _ _ _ _ _ _ _ w785 _] -> w213
      tunnel: [_ _ _ _ _ _ _ _ _ _ w784 _] -> w212
      frame #0 {
        # "Refining the Left and Right Image Acquisition Process:\n\nLoading the images.\nResizing the images to match the grid image size"
        n93 = Build Array(w232, w233) -> (w241:string[])
        n94 = Index Array(array=w231, index #1=0 ("index"), index #2=1 ("index")) -> (element #1=w240:T2, element #2=w239:T2)
        n95 = Build Array(w240, w239) -> (w238:T2[])
        n96 = local read "Grid Y"() -> (w242:i32)
        n97 = local read "Grid X"() -> (w243:i32)
        n98 = for {
          tunnel: w243 -> [w254]
          tunnel: w242 -> [w253]
          tunnel: w230 -> [w252]
          tunnel: w241 -> [w250] mode=indexing
          tunnel: w238 -> [w249] mode=indexing
          tunnel: [w248] -> w237 mode=indexing
          tunnel: w234 -> [w246]
          n99 = Build Path(base path=w246, name or relative path=w250) -> (appended path=w251:path)
          n100 = call "IMAQ ReadFile"("File Path"=w251, "Image"=w249) -> ("Image Out"=w247:T2)  [unwired: 3 in, 6 out]
          n101 = call "IMAQ Resample"("X Resolution"=w254, "Y Resolution"=w253, "Interpolation Type"=w252, "Image Dst"=w247, "Image Src"=w247) -> ("Image Dst Out"=w248:T2)  [unwired: 5 in, 1 out]
        }
        n102 = Index Array(array=w237) -> (element #1=→"Left Sample":T2, element #2=→"Right Sample":T2)  [unwired: 2 in]
      }
      frame #1 {
        # "Initiating time measurement for the system process."
        n103 = Get Date/Time In Seconds() -> (seconds since 1Jan1904=w256:timestamp)
        n104 = To Double Precision Float(number=w256) -> (double precision float=→"Start Time":dbl)
      }
      frame #2 {
        # "barrel Distortion Correction Process:\n\nTransferring calibration information on the captured images.\nRectifying lens distortion for both the left and right images"
        n105 = Index Array(array=w258, index #1=2 ("index"), index #2=3 ("index")) -> (element #1=w262:T2, element #2=w261:T2)
        n106 = Build Array(w262, w261) -> (w260:T2[])
        n107 = local read "Right Sample"() -> (w266:T2)
        n108 = local read "Left Sample"() -> (w267:T2)
        n109 = Build Array(w267, w266) -> (w265:T2[])
        n110 = for {
          tunnel: w265 -> [w270] mode=indexing
          tunnel: [w271] -> w259 mode=indexing
          tunnel: w260 -> [w269] mode=indexing
          tunnel: w257 -> [w268]
          n111 = call "IMAQ Set Calibration Info"("Image Dst"=w270, "Image Src"=w268) -> ("Calibrated Image"=w272:T2)  [unwired: 8 in, 1 out]
          n112 = call "IMAQ Correct Calibrated Image"("Image Dst"=w269, "Image Src"=w272) -> ("Corrected Image"=w271:T2)  [unwired: 8 in, 1 out]
        }
        "corrected" <- w259
      }
      frame #3 {
        # "Measuring the elapsed time for the barrel distortion correction process."
        n113 = local read "Start Time"() -> (w274:dbl)
        n114 = Get Date/Time In Seconds() -> (seconds since 1Jan1904=w276:timestamp)
        n115 = To Double Precision Float(number=w276) -> (double precision float=w275:dbl)
        "Correction End Time" <- w275
        n116 = Subtract(x=w275, y=w274) -> (x-y=→"Correction":dbl)
      }
      frame #4 {
        w285 = 0 items=["Polynomial"] ("Model")
        w282 = 0 items=["Polynomial", "Background Correction", "NiBlack"] ("Method")
        w293 = 5 ("Window Size")
        w314 = 5 items=["Red", "Green", "Blue", "Hue", "Saturation", "Luminance", "Value", "Intensity"] ("Color Plane")
        # "Flat Fielding Process:\n\nExtracting luminance planes for both images.\nMeasuring the SSIM factor.\nAveraging the luminance planes.\nEstimating the Master Flat Field plane.\nGenerating the flat-fielded planes.\nMeasuring the SSIM of the flat-fielded planes.\nReplacing the planes with the higher SSIM."
        n117 = Index Array(array=w292, index #1=9 ("index"), index #7=15 ("index")) -> (element #1=w312:T2, element #2=w311:T2, element #3=w309:T2, element #4=w303:T2, element #5=w302:T2, element #6=w299:T2, element #7=w298:T2)  [unwired: 5 in]
        n118 = local read "corrected"() -> (w287:T2[])
        n119 = Build Array(w312, w311) -> (w310:T2[])
        n120 = Build Array(w303, w302) -> (w301:T2[])
        n121 = Build Array(w299, w298) -> (w297:T2[])
        n122 = local read "corrected size"() -> (w277:cluster{"X Resolution":i32, "Y Resolution":i32})
        n123 = for {
          tunnel: w314 -> [w330]
          tunnel: w287 -> [w329] mode=indexing
          tunnel: w310 -> [w328] mode=indexing
          tunnel: [w327] -> w306 mode=indexing
          tunnel: [w327] -> w286 mode=indexing
          n124 = call "IMAQ ExtractSingleColorPlane"("Color Plane"=w330, "Image Dst"=w328, "Image Src"=w329) -> ("Image Dst Out"=w327:T2)  [unwired: 7 in, 1 out]
        }
        n125 = Bundle("Model"=w285, "corrected size"=w277, "Polynomial Degree"=1) -> (w278:T12)  [unwired: 1 in]
        n126 = Bundle("Estimate Background?"=TRUE, "Method"=w282, "Polynomial Degree"=1, "corrected size"=w277, "Niblack Deviation Factor (0.2)"=0.2) -> (w279:T13)  [unwired: 1 in]
        n127 = call "IMAQ Compute Average Image"("Image Dst"=w309, "Images"=w306) -> ("Image Dst Out"=w294:T2)  [unwired: 8 in, 1 out]
        n128 = Index Array(array=w286) -> (element #1=w308:T2, element #2=w307:T2)  [unwired: 2 in]
        n129 = for {
          tunnel: w286 -> [w324] mode=indexing
          tunnel: w294 -> [w326]
          tunnel: [w325] -> w290 mode=indexing
          tunnel: w301 -> [w322] mode=indexing
          tunnel: w297 -> [w321] mode=indexing
          tunnel: w278 -> [w320]
          tunnel: w279 -> [w319]
          n130 = call "IMAQ Estimate Flat Field Model"("Image Src"=w324, "Image Dst"=w322, "Mask Image"=w326, "Surface Fit Options"=w320, "Background Estimation Options"=w319) -> ("Flat Field Image Out"=w323:T2)  [unwired: 9 in, 1 out]
          n131 = call "IMAQ Flat Field Correction"("Image Src"=w324, "Image Dst"=w321, "Flat Field Image"=w323) -> ("Corrected Image"=w325:T2)  [unwired: 10 in, 2 out]
        }
        n132 = call-poly "IMAQ SSIM"("Window Size"=w293, "Reference Image"=w307, "Test Image"=w308) -> ("Mean SSIM"=w296:dbl)  [unwired: 4 in, 4 out]
        "SSIM Original" <- w296
        n133 = Index Array(array=w290) -> (element #1=w305:T2, element #2=w304:T2)  [unwired: 2 in]
        n134 = call-poly "IMAQ SSIM"("Window Size"=w293, "Reference Image"=w304, "Test Image"=w305) -> ("Mean SSIM"=w295:dbl)  [unwired: 4 in, 4 out]
        "SSIM Flat" <- w295
        n135 = Greater?(x=w296, y=w295) -> (0:w291:bool)
        "Original Luma?" <- w291
        n136 = Select(t=w286, s=w291, f=w290) -> (s? t:f=w289:T2[])
        n137 = for {
          tunnel: [w318] -> w288 mode=indexing
          tunnel: w287 -> [w317] mode=indexing
          tunnel: w289 -> [w316] mode=indexing
          w315 = u16 1 items=["RGB", "HSL", "HSV", "HSI"] ("Color Mode")
          n138 = call "IMAQ ReplaceColorPlane"("Image Src"=w317, "Color Mode"=w315, "Blue or Luma or Val or Inten Plane"=w316) -> ("Image Dst Out"=w318:T2)  [unwired: 11 in, 1 out]
        }
        "Adjusted" <- w288
      }
      frame #5 {
        # "Measuring the elapsed time for the Flat-Fielding process."
        n139 = local read "Correction End Time"() -> (w332:dbl)
        n140 = Get Date/Time In Seconds() -> (seconds since 1Jan1904=w334:timestamp)
        n141 = To Double Precision Float(number=w334) -> (double precision float=w333:dbl)
        "Flat Fielding End Time" <- w333
        n142 = Subtract(x=w333, y=w332) -> (x-y=→"Flat Fielding":dbl)
      }
      frame #6 {
        # "Image Wrapping:\n\nProjecting both the left and right images using the updated coordinates."
        n143 = Build Array(w335, w336) -> (w340:T2[])
        n144 = local read "Adjusted"() -> (w341:T2[])
        n145 = for {
          tunnel: w341 -> [w342] mode=indexing
          tunnel: w340 -> [w344] mode=indexing
          tunnel: [w343] -> w337 mode=indexing
          n146 = call "IMAQ Set Calibration Info"("Image Dst"=w342, "Image Src"=w344) -> ("Calibrated Image"=w345:T2)  [unwired: 8 in, 1 out]
          n147 = call "IMAQ Correct Calibrated Image"("Image Dst"=w342, "Image Src"=w345) -> ("Corrected Image"=w343:T2)  [unwired: 8 in, 1 out]
        }
        "Wrapped" <- w337
        n148 = Index Array(array=w337) -> (element #1=→"Left corrected, adjusted, and wrapped image":T2, element #2=→"Right corrected, adjusted, and wrapped image":T2)  [unwired: 2 in]
      }
      frame #7 {
        w381 = 0
        # "Region of Interest Extraction:\n\nIdentifying the ROIs in both left and right images.\nExtracting the RGB planes within the defined ROIs."
        n149 = Index Array(array=w351, index #1=4 ("index"), index #2=5 ("index")) -> (element #1=w372:T2, element #2=w371:T2)
        n150 = Build Array(w372, w371) -> (w370:T2[])
        n151 = local read "ROI_X"() -> (w348:i32)
        n152 = local read "Wrapped X"() -> (w346:i32)
        n153 = local read "Wrapped Y"() -> (w347:i32)
        n154 = Subtract(x=w346, y=w348) -> (x-y=w380:i32)
        n155 = Build Array(w381, w381, w348, w347) -> (w377:i32[])
        n156 = Build Array(w380, 0 ("element"), w346, w347) -> (w378:i32[])
        n157 = local read "Wrapped"() -> (w376:T2[])
        n158 = Build Array(w378, w377) -> (w375:i32[][])
        n159 = for {
          tunnel: w375 -> [w385] mode=indexing
          tunnel: [w382] -> _ mode=indexing
          tunnel: [w384] -> w354 mode=indexing
          tunnel: w370 -> [w383] mode=indexing
          tunnel: w376 -> [w382] mode=indexing
          n160 = call "IMAQ ColorImageToArray"("Optional Rectangle"=w385, "Image"=w382) -> ("Image Pixels (U32)"=w386:u32[][])  [unwired: 2 in, 2 out]
          n161 = call "IMAQ ArrayToColorImage"("Image Pixels (U32)"=w386, "Image"=w383) -> ("Image Out"=w384:T2)  [unwired: 3 in, 1 out]
        }
        n162 = Index Array(array=w354) -> (element #1=w356:T2, element #2=w355:T2)  [unwired: 2 in]
        "ROI_R" <- w355
        "ROI_L" <- w356
        n163 = Index Array(array=w350, index #1=16 ("index"), index #6=21 ("index")) -> (element #1=w368:T2, element #2=w367:T2, element #3=w366:T2, element #4=w365:T2, element #5=w364:T2, element #6=w363:T2)  [unwired: 4 in]
        n164 = call "IMAQ ExtractColorPlanes"("Blue or Luma or Val or Inten Plane"=w366, "Green or Sat Plane"=w367, "Red or Hue Plane"=w368, "Image Src"=w356) -> ("Blue or Luma or Val or Inten Plane out"=w360:T2, "Green or Sat Plane out"=w361:T2, "Red or Hue Plane out"=w362:T2)  [unwired: 4 in, 1 out]
        n165 = Build Array(w362, w361, w360) -> (→"RGB Left":T2[])
        n166 = call "IMAQ ExtractColorPlanes"("Blue or Luma or Val or Inten Plane"=w363, "Green or Sat Plane"=w364, "Red or Hue Plane"=w365, "Image Src"=w355) -> ("Blue or Luma or Val or Inten Plane out"=w357:T2, "Green or Sat Plane out"=w358:T2, "Red or Hue Plane out"=w359:T2)  [unwired: 4 in, 1 out]
        n167 = Build Array(w359, w358, w357) -> (→"RGB Right":T2[])
      }
      frame #8 {
        # "Blending the Regions Of Interest (ROIs) based on the chosen method."
        n168 = case shown="\"MBB\"" "Blending Method" {
          tunnel: w396 -> [w401 w466 w734]
          tunnel: w395 -> [w402 w465 w733]
          tunnel: w394 -> [w400 _ _]
          tunnel: w393 -> [w399 _ _]
          tunnel: w392 -> [_ w464 _]
          tunnel: w391 -> [_ w463 _]
          tunnel: w390 -> [_ w462 _]
          tunnel: [w398 w461 w732] -> w389
          tunnel: w388 -> [_ w460 _]
          tunnel: w387 -> [_ w459 _]
          frame "WA" {
            n169 = stacked-sequence {
              tunnel: w402 -> [w417]
              tunnel: w401 -> [w412]
              tunnel: w400 -> [w406]
              tunnel: w399 -> [w405]
              tunnel: [w413] -> w398
              frame #0 {
                # "Weighted Average Blending:\n\nComputing the weighted ROIs.\nCombining the weighted ROIs.\nAveraging the combined ROIs."
                n170 = call-poly <vilib>:"IMAQ ImageToEDVR.vi"("Image"=w405) -> ("EDVR 2D SGL"=w425:refnum<data-value>)  [unwired: 8 in, 2 out]
                n171 = Index Array(array=w412, index #1=22 ("index")) -> (element #1=w411:T2, element #2=w410:T2, element #3=w409:T2)  [unwired: 2 in]
                n172 = local read "RGB Right"() -> (w422:T2[])
                n173 = local read "RGB Left"() -> (w423:T2[])
                n174 = Build Array(w411, w410, w409) -> (w408:T2[])
                n175 = call-poly <vilib>:"IMAQ ImageToEDVR.vi"("Image"=w406) -> ("EDVR 2D SGL"=w424:refnum<data-value>)  [unwired: 8 in, 2 out]
                n176 = for {
                  tunnel: w422 -> [w434] mode=indexing
                  tunnel: w423 -> [w427] mode=indexing
                  tunnel: w424 -> [w432]
                  tunnel: w425 -> [w431]
                  tunnel: [w428] -> w421 mode=indexing
                  tunnel: w408 -> [w426] mode=indexing
                  n177 = call-poly <vilib>:"IMAQ ImageToEDVR.vi"("Image"=w434) -> ("EDVR 2D U8"=w435:refnum<data-value>)  [unwired: 8 in, 2 out]
                  n178 = call-poly <vilib>:"IMAQ ImageToEDVR.vi"("Image"=w427) -> ("EDVR 2D U8"=w433:refnum<data-value>)  [unwired: 8 in, 2 out]
                  n179 = in-place {
                    in-place-border: [w443] -> _
                    in-place-border: [w438] -> _
                    in-place-border: [w437] -> _
                    in-place-border: [w436] -> w429
                    n180 = in-place-dvr #1(w432) -> (w439:sgl[][])  [unwired: 1 out]
                    n181 = in-place-dvr #2(w431) -> (w440:sgl[][])  [unwired: 1 out]
                    n182 = in-place-dvr #3(w435) -> (w441:u8[][])  [unwired: 1 out]
                    n183 = in-place-dvr #4(w433) -> (w442:u8[][])  [unwired: 1 out]
                    n184 = for {
                      tunnel: w441 -> [w451] mode=indexing
                      workers-P: _ -> [_]
                      tunnel: [w450] -> w443 mode=indexing
                      tunnel: w442 -> [w449] mode=indexing
                      tunnel: w440 -> [w448] mode=indexing
                      tunnel: w439 -> [w447] mode=indexing
                      tunnel: [w446] -> w438 mode=indexing
                      tunnel: [w445] -> w437 mode=indexing
                      tunnel: [w444] -> w436 mode=indexing
                      n185 = for {
                        tunnel: w451 -> [w458] mode=indexing
                        tunnel: [w454] -> w450 mode=indexing
                        tunnel: w449 -> [w452] mode=indexing
                        tunnel: w447 -> [w453] mode=indexing
                        tunnel: w448 -> [w457] mode=indexing
                        tunnel: [w456] -> w446 mode=indexing
                        tunnel: [w455] -> w444 mode=indexing
                        tunnel: [w454] -> w445 mode=indexing
                        n186 = Multiply(x=w452, y=w453) -> (x*y=w456:sgl)
                        n187 = Multiply(x=w458, y=w457) -> (x*y=w454:sgl)
                        n188 = Add(x=w454, y=w456) -> (x+y=w455:sgl)
                      }
                    }
                    n189 = in-place-dvr #1(w439) -> ()  [unwired: 2 out]
                    n190 = in-place-dvr #2(w440) -> ()  [unwired: 2 out]
                    n191 = in-place-dvr #3(w441) -> ()  [unwired: 2 out]
                    n192 = in-place-dvr #4(w442) -> ()  [unwired: 2 out]
                  }
                  n193 = To Unsigned Byte Integer(number=w429) -> (unsigned 8bit integer=w430:u8[][])
                  n194 = call "IMAQ ArrayToImage"("Image Pixels (U8)"=w430, "Image"=w426) -> ("Image Out"=w428:T2)  [unwired: 8 in, 1 out]
                }
                n195 = local read "ROI_X"() -> (w403:i32)
                n196 = local read "Wrapped Y"() -> (w404:i32)
                n197 = Index Array(array=w417, index=6) -> (element=w415:T2)
                n198 = call "IMAQ SetImageSize"("Y Resolution"=w404, "X Resolution"=w403, "Image"=w415) -> ("Image Out"=w414:T2)  [unwired: 2 in, 1 out]
                n199 = Index Array(array=w421) -> (element #1=w420:T2, element #2=w419:T2, element #3=w418:T2)  [unwired: 3 in]
                n200 = call "IMAQ ReplaceColorPlane"("Image Src"=w414, "Red or Hue Plane"=w420, "Green or Sat Plane"=w419, "Blue or Luma or Val or Inten Plane"=w418) -> ("Image Dst Out"=w413:T2)  [unwired: 10 in, 1 out]
              }
            }
          }
          frame "MBB" {
            n201 = stacked-sequence {
              tunnel: w466 -> [w470 w496 w546 _ w658 w699]
              tunnel: w465 -> [_ _ _ w608 w659 w697]
              tunnel: w464 -> [_ w495 w548 _ _ w698]
              tunnel: w463 -> [_ w494 _ _ _ _]
              tunnel: w462 -> [_ _ w547 _ _ _]
              tunnel: [_ _ _ _ _ w696] -> w461
              tunnel: w460 -> [w468 _ _ _ _ _]
              tunnel: w459 -> [w469 _ _ _ _ _]
              frame #0 {
                # "Multi-Band Blending:\n\nMasking the ROIs.\nGenerating the Gaussian Pyramid of the masked ROIs.\nGenerating the Laplacian Pyramid of the ROIs.\nBlending the Pyramids starting from the lowest resolution."
                n202 = Index Array(array=w470, index #1=25 ("index"), index #6=30 ("index")) -> (element #1=w481:T2, element #2=w480:T2, element #3=w479:T2, element #4=w477:T2, element #5=w476:T2, element #6=w475:T2)  [unwired: 4 in]
                n203 = local read "RGB Right"() -> (w471:T2[])
                n204 = local read "RGB Left"() -> (w472:T2[])
                n205 = Build Array(w481, w480, w479) -> (w478:T2[])
                n206 = Build Array(w477, w476, w475) -> (w474:T2[])
                n207 = for {
                  tunnel: w472 -> [w491] mode=indexing
                  tunnel: w471 -> [w490] mode=indexing
                  tunnel: [w489] -> w483 mode=indexing
                  tunnel: [w488] -> w482 mode=indexing
                  tunnel: w478 -> [w487] mode=indexing
                  tunnel: w474 -> [w486] mode=indexing
                  tunnel: w469 -> [w485]
                  tunnel: w468 -> [w484]
                  n208 = call "IMAQ Multiply"("Image Src A"=w490, "Image Dst"=w486, "Image Src B"=w484) -> ("Image Dst Out"=w489:T2)  [unwired: 4 in, 1 out]
                  n209 = call "IMAQ Multiply"("Image Src A"=w491, "Image Dst"=w487, "Image Src B"=w485) -> ("Image Dst Out"=w488:T2)  [unwired: 4 in, 1 out]
                }
                "Masked RGB Right MBB" <- w483
                "Masked RGB Left MBB" <- w482
              }
              frame #1 {
                w507 = 6 ("length")
                w514 = 31 ("index")
                n210 = Array Subset(array=w496, index=w514, length=w507) -> (w518:T2[])
                n211 = Add(x=w514, y=w507) -> (x+y=w513:i32)
                n212 = Array Subset(array=w496, index=w513, length=w507) -> (w517:T2[])
                n213 = Add(x=w513, y=w507) -> (x+y=w512:i32)
                n214 = Array Subset(array=w496, index=w512, length=w507) -> (w516:T2[])
                n215 = Add(x=w512, y=w507) -> (x+y=w511:i32)
                n216 = Array Subset(array=w496, index=w511, length=w507) -> (w515:T2[])
                n217 = Add(x=w511, y=w507) -> (x+y=w510:i32)
                n218 = Array Subset(array=w496, index=w510, length=w507) -> (w505:T2[])
                n219 = Add(x=w510, y=w507) -> (x+y=w509:i32)
                n220 = Array Subset(array=w496, index=w509, length=w507) -> (w504:T2[])
                n221 = Add(x=w509, y=w507) -> (x+y=w508:i32)
                n222 = local read "Wrapped X"() -> (w492:i32)
                n223 = local read "Wrapped Y"() -> (w493:i32)
                n224 = Add(x=w508, y=w507) -> (x+y=w506:i32)
                n225 = Array Subset(array=w496, index=w508, length=w507) -> (w503:T2[])
                n226 = local read "Masked RGB Right MBB"() -> (w499:T2[])
                n227 = local read "Masked RGB Left MBB"() -> (w500:T2[])
                n228 = local read "Y0"() -> (w523:dbl)
                n229 = local read "Y1"() -> (w522:dbl)
                n230 = local read "Y2"() -> (w521:dbl)
                n231 = local read "X0"() -> (w526:dbl)
                n232 = local read "X1"() -> (w525:dbl)
                n233 = local read "X2"() -> (w524:dbl)
                n234 = Array Subset(array=w496, index=w506, length=w507) -> (w502:T2[])
                n235 = Build Array(w493, w523, w522, w521) -> (w519:dbl[])
                n236 = Build Array(w492, w526, w525, w524) -> (w520:dbl[])
                n237 = Build Array(w518, w517, w516, w515, w505, w504, w503, w502) -> (w501:T2[][])
                n238 = Insert Into Array(array=w500, new element=w499) -> (w498:T2[])  [unwired: 1 in]
                n239 = for {
                  tunnel: w520 -> [w534] mode=indexing
                  tunnel: w519 -> [w533] mode=indexing
                  tunnel: [w532] -> w497 mode=indexing
                  tunnel: w494 -> [w531]
                  tunnel: w501 -> [w529] mode=indexing
                  tunnel: w495 -> [w527]
                  tunnel: w498 -> [w528]
                  n240 = for {
                    N: 6 -> [_]
                    tunnel: w528 -> [w542] mode=indexing
                    tunnel: w534 -> [w541]
                    tunnel: w533 -> [w540]
                    tunnel: [w539] -> w532 mode=indexing
                    tunnel: w531 -> [w538]
                    tunnel: w529 -> [w537] mode=indexing
                    tunnel: w527 -> [w535]
                    n241 = call "IMAQ Convolute"("Kernel"=w538, "Image Src"=w542) -> ("error out"=w543:errorcluster, "Image Dst Out"=w536:T2)  [unwired: 8 in]
                    n242 = call "IMAQ Resample"("X Resolution"=w541, "Y Resolution"=w540, "error in (no error)"=w543, "Interpolation Type"=w535, "Image Dst"=w537, "Image Src"=w536) -> ("Image Dst Out"=w539:T2)  [unwired: 4 in, 1 out]
                  }
                }
                "GP" <- w497
              }
              frame #2 {
                w565 = 6 ("length")
                w572 = 55 ("index")
                n243 = Array Subset(array=w546, index=w572, length=w565) -> (w576:T2[])
                n244 = Add(x=w572, y=w565) -> (x+y=w571:i32)
                n245 = Array Subset(array=w546, index=w571, length=w565) -> (w575:T2[])
                n246 = Add(x=w571, y=w565) -> (x+y=w570:i32)
                n247 = Array Subset(array=w546, index=w570, length=w565) -> (w574:T2[])
                n248 = Add(x=w570, y=w565) -> (x+y=w569:i32)
                n249 = Array Subset(array=w546, index=w569, length=w565) -> (w573:T2[])
                n250 = Add(x=w569, y=w565) -> (x+y=w568:i32)
                n251 = Array Subset(array=w546, index=w568, length=w565) -> (w563:T2[])
                n252 = Add(x=w568, y=w565) -> (x+y=w567:i32)
                n253 = local read "ROI_X"() -> (w545:i32)
                n254 = local read "Wrapped Y"() -> (w544:i32)
                n255 = Array Subset(array=w546, index=w567, length=w565) -> (w562:T2[])
                n256 = Add(x=w567, y=w565) -> (x+y=w566:i32)
                n257 = local read "X0"() -> (w580:dbl)
                n258 = local read "X1"() -> (w579:dbl)
                n259 = local read "Y0"() -> (w578:dbl)
                n260 = local read "Y1"() -> (w577:dbl)
                n261 = Add(x=w566, y=w565) -> (x+y=w564:i32)
                n262 = Array Subset(array=w546, index=w566, length=w565) -> (w561:T2[])
                n263 = Build Array(w544, w578, w577) -> (w555:dbl[])
                n264 = Build Array(w545, w580, w579) -> (w557:dbl[])
                n265 = local read "GP"() -> (w553:T2[][])
                n266 = Array Subset(array=w546, index=w564, length=w565) -> (w560:T2[])
                n267 = Reshape Array(w553, 24 ("dimension size")) -> (w552:T2[])
                n268 = Build Array(w576, w575, w574, w573, w563, w562, w561, w560) -> (w559:T2[][])
                n269 = Reverse 1D Array(array=w557) -> (reversed array=w556:dbl[])
                n270 = Reverse 1D Array(array=w555) -> (reversed array=w554:dbl[])
                n271 = Reverse 1D Array(array=w552) -> (reversed array=w551:T2[])
                n272 = for {
                  tunnel: w556 -> [w589] mode=indexing
                  tunnel: w554 -> [w588] mode=indexing
                  tunnel: [w587] -> w558 mode=indexing
                  tunnel: w547 -> [w586]
                  tunnel: w559 -> [w584] mode=indexing
                  tunnel: w548 -> [w583]
                  tunnel: w551 -> [w582]
                  tunnel: sgl 15.0 ("Divider (kernel sum)") -> [w581]
                  n273 = for {
                    N: 6 -> [_]
                    tunnel: w582 -> [w594] mode=indexing
                    tunnel: w589 -> [w598]
                    tunnel: w588 -> [w597]
                    tunnel: [w592] -> w587 mode=indexing
                    tunnel: w586 -> [w591]
                    tunnel: w584 -> [w596] mode=indexing
                    tunnel: w583 -> [w595]
                    tunnel: w581 -> [w590]
                    n274 = call "IMAQ Resample"("X Resolution"=w598, "Y Resolution"=w597, "Interpolation Type"=w595, "Image Dst"=w596, "Image Src"=w594) -> ("Image Dst Out"=w593:T2)  [unwired: 5 in, 1 out]
                    n275 = call "IMAQ Convolute"("Kernel"=w591, "Divider (kernel sum)"=w590, "Image Src"=w593) -> ("Image Dst Out"=w592:T2)  [unwired: 7 in, 1 out]
                  }
                }
                "LP" <- w558
              }
              frame #3 {
                n276 = local read "GP"() -> (w624:T2[][])
                n277 = local read "LP"() -> (w638:T2[][])
                n278 = Array Subset(array=w638, index (row)=0 ("index"), length (row)=3 ("length"), index (col)=0 ("index"), length (col)=3 ("length")) -> (w630:T2[][])
                n279 = Array Subset(array=w638, index (row)=0 ("index"), length (row)=3 ("length"), index (col)=3 ("index"), length (col)=3 ("length")) -> (w629:T2[][])
                n280 = Array Subset(array=w624, index (row)=0 ("index"), length (row)=3 ("length"), index (col)=0 ("index"), length (col)=3 ("length")) -> (w619:T2[][])
                n281 = Array Subset(array=w624, index (row)=0 ("index"), length (row)=3 ("length"), index (col)=3 ("index"), length (col)=3 ("length")) -> (w618:T2[][])
                n282 = for {
                  tunnel: w630 -> [w651] mode=indexing
                  tunnel: w629 -> [w650] mode=indexing
                  tunnel: [w646] -> w614 mode=indexing
                  tunnel: w619 -> [w649] mode=indexing
                  tunnel: w618 -> [w648] mode=indexing
                  tunnel: [w647] -> w607 mode=indexing
                  n283 = for {
                    tunnel: w651 -> [w657] mode=indexing
                    tunnel: w650 -> [w656] mode=indexing
                    tunnel: [w655] -> w647 mode=indexing
                    tunnel: w649 -> [w654] mode=indexing
                    tunnel: w648 -> [w653] mode=indexing
                    tunnel: [w652] -> w646 mode=indexing
                    n284 = call "IMAQ Add"("Image Src A"=w657, "Image Src B"=w656) -> ("Image Dst Out"=w655:T2)  [unwired: 5 in, 1 out]
                    n285 = call "IMAQ Add"("Image Src A"=w654, "Image Src B"=w653) -> ("Image Dst Out"=w652:T2)  [unwired: 5 in, 1 out]
                  }
                }
                "Combined Laplace" <- w607
                n286 = Array Subset(array=w607, index (row)=0 ("index"), length (row)=3 ("length")) -> (w613:T2[][])  [unwired: 2 in]
                n287 = Array Subset(array=w614, index (row)=2 ("index")) -> (w612:T2[][])  [unwired: 3 in]
                n288 = for {
                  tunnel: w613 -> [w642] mode=indexing
                  tunnel: w612 -> [w641] mode=indexing
                  tunnel: [w640] -> w610 mode=indexing
                  n289 = for {
                    tunnel: w642 -> [w645] mode=indexing
                    tunnel: w641 -> [w644] mode=indexing
                    tunnel: [w643] -> w640 mode=indexing
                    n290 = call "IMAQ Add"("Image Src A"=w645, "Image Src B"=w644) -> ("Image Dst Out"=w643:T2)  [unwired: 5 in, 1 out]
                  }
                }
                n291 = Index Array(array=w608, index=7) -> (element=w606:T2)
                n292 = local read "X1"() -> (w600:dbl)
                n293 = local read "Y1"() -> (w599:dbl)
                n294 = Reshape Array(w610, 3 ("dimension size")) -> (w601:T2[])
                n295 = call "IMAQ SetImageSize"("Y Resolution"=w599, "X Resolution"=w600, "Image"=w606) -> ("Image Out"=w605:T2)  [unwired: 2 in, 1 out]
                n296 = Index Array(array=w601) -> (element #1=w604:T2, element #2=w603:T2, element #3=w602:T2)  [unwired: 3 in]
                n297 = call "IMAQ ReplaceColorPlane"("Image Src"=w605, "Red or Hue Plane"=w604, "Green or Sat Plane"=w603, "Blue or Luma or Val or Inten Plane"=w602) -> ()  [unwired: 10 in, 2 out]
              }
              frame #4 {
                w678 = u16 0 items=["RGB", "HSL", "HSV", "HSI"] ("Color Mode")
                n298 = Index Array(array=w658, index #1=80 ("index")) -> (element #1=w681:T2, element #2=w680:T2, element #3=w679:T2)  [unwired: 2 in]
                n299 = Index Array(array=w659, index=7) -> (element=w660:T2)
                n300 = local read "Combined Laplace"() -> (w677:T2[][])
                n301 = call "IMAQ ExtractColorPlanes"("Blue or Luma or Val or Inten Plane"=w679, "Color Mode"=w678, "Green or Sat Plane"=w680, "Red or Hue Plane"=w681, "Image Src"=w660) -> ("Blue or Luma or Val or Inten Plane out"=w684:T2, "Green or Sat Plane out"=w685:T2, "Red or Hue Plane out"=w686:T2)  [unwired: 3 in, 1 out]
                n302 = local read "Correction Interpolation"() -> (w662:u32)
                n303 = Array Subset(array=w677, index (row)=1 ("index"), length (row)=1 ("length")) -> (w674:T2[][])  [unwired: 2 in]
                n304 = Build Array(w686, w685, w684) -> (w683:T2[])
                n305 = local read "X0"() -> (w669:dbl)
                n306 = local read "Y0"() -> (w668:dbl)
                n307 = Index Array(array=w659, index=8) -> (element=w670:T2)
                n308 = Reshape Array(w674, 3 ("dimension size")) -> (w672:T2[])
                n309 = for {
                  tunnel: w683 -> [w691] mode=indexing
                  tunnel: w669 -> [w693]
                  tunnel: w668 -> [w692]
                  tunnel: [w688] -> w666 mode=indexing
                  tunnel: w672 -> [w689] mode=indexing
                  tunnel: w662 -> [w687]
                  n310 = call "IMAQ Resample"("X Resolution"=w693, "Y Resolution"=w692, "Interpolation Type"=w687, "Image Src"=w691) -> ("Image Dst Out"=w690:T2)  [unwired: 6 in, 1 out]
                  n311 = call "IMAQ Add"("Image Src A"=w690, "Image Src B"=w689) -> ("Image Dst Out"=w688:T2)  [unwired: 5 in, 1 out]
                }
                n312 = call "IMAQ SetImageSize"("Y Resolution"=w668, "X Resolution"=w669, "Image"=w670) -> ("Image Out"=w667:T2)  [unwired: 2 in, 1 out]
                n313 = Index Array(array=w666) -> (element #1=w663:T2, element #2=w664:T2, element #3=w665:T2)  [unwired: 3 in]
                n314 = call "IMAQ ReplaceColorPlane"("Image Src"=w667, "Red or Hue Plane"=w663, "Green or Sat Plane"=w664, "Blue or Luma or Val or Inten Plane"=w665) -> ()  [unwired: 10 in, 2 out]
              }
              frame #5 {
                w715 = u16 0 items=["RGB", "HSL", "HSV", "HSI"] ("Color Mode")
                n315 = Index Array(array=w699, index #1=83 ("index")) -> (element #1=w718:T2, element #2=w717:T2, element #3=w716:T2)  [unwired: 2 in]
                n316 = Index Array(array=w697, index=8) -> (element=w700:T2)
                n317 = local read "Combined Laplace"() -> (w714:T2[][])
                n318 = call "IMAQ ExtractColorPlanes"("Blue or Luma or Val or Inten Plane"=w716, "Color Mode"=w715, "Green or Sat Plane"=w717, "Red or Hue Plane"=w718, "Image Src"=w700) -> ("Blue or Luma or Val or Inten Plane out"=w721:T2, "Green or Sat Plane out"=w722:T2, "Red or Hue Plane out"=w723:T2)  [unwired: 3 in, 1 out]
                n319 = Array Subset(array=w714, index (row)=2 ("index"), length (row)=1 ("length")) -> (w711:T2[][])  [unwired: 2 in]
                n320 = local read "ROI_X"() -> (w695:i32)
                n321 = local read "Wrapped Y"() -> (w694:i32)
                n322 = Build Array(w723, w722, w721) -> (w720:T2[])
                n323 = Index Array(array=w697, index=9) -> (element=w707:T2)
                n324 = Reshape Array(w711, 3 ("dimension size")) -> (w709:T2[])
                n325 = for {
                  tunnel: w720 -> [w729] mode=indexing
                  tunnel: w695 -> [w730]
                  tunnel: w694 -> [w724]
                  tunnel: [w728] -> w702 mode=indexing
                  tunnel: w709 -> [w726] mode=indexing
                  tunnel: w698 -> [w725]
                  tunnel: w695 -> [_]
                  n326 = call "IMAQ Resample"("X Resolution"=w730, "Y Resolution"=w724, "Interpolation Type"=w725, "Image Src"=w729) -> ("Image Dst Out"=w727:T2)  [unwired: 6 in, 1 out]
                  n327 = call "IMAQ Add"("Image Src A"=w727, "Image Dst"=w726, "Image Src B"=w726) -> ("Image Dst Out"=w728:T2)  [unwired: 4 in, 1 out]
                }
                n328 = call "IMAQ SetImageSize"("Y Resolution"=w694, "X Resolution"=w695, "Image"=w707) -> ("Image Out"=w706:T2)  [unwired: 2 in, 1 out]
                n329 = Index Array(array=w702) -> (element #1=w703:T2, element #2=w704:T2, element #3=w705:T2)  [unwired: 3 in]
                n330 = call "IMAQ ReplaceColorPlane"("Image Src"=w706, "Red or Hue Plane"=w703, "Green or Sat Plane"=w704, "Blue or Luma or Val or Inten Plane"=w705) -> ("Image Dst Out"=w696:T2)  [unwired: 10 in, 1 out]
              }
            }
          }
          frame "WE" {
            w737 = u16 0 items=["RGB", "HSL", "HSV", "HSI"] ("Color Mode")
            # "Wavelet Extraction Blending:\n\nApplying the Haar filter on the ROIs.\nExtracting the low frequencies.\nCombining and scaling the low frequencies of the ROIs."
            n331 = Index Array(array=w734, index #1=86 ("index")) -> (element #1=w747:T2, element #2=w746:T2, element #3=w745:T2)  [unwired: 2 in]
            n332 = local read "Original Luma?"() -> (w748:bool)
            n333 = Build Array(w747, w746, w745) -> (w752:T2[])
            n334 = case shown="True" w748 {
              tunnel: [w754 w758] -> w749
              frame False {
                n335 = local read "SSIM Flat"() -> (w757:dbl)
                n336 = Multiply(x=w757, y=10.0) -> (x*y=w755:dbl)
                n337 = Round Toward +Infinity(x=w755) -> (ceil(x): smallest int >= x=w754:dbl)
              }
              frame True {
                n338 = local read "SSIM Original"() -> (w761:dbl)
                n339 = Multiply(x=w761, y=10.0) -> (x*y=w759:dbl)
                n340 = Round Toward +Infinity(x=w759) -> (ceil(x): smallest int >= x=w758:dbl)
              }
            }
            n341 = local read "RGB Right"() -> (w751:T2[])
            n342 = local read "RGB Left"() -> (w750:T2[])
            n343 = for {
              tunnel: w752 -> [w774] mode=indexing
              tunnel: [w762] -> w740
              tunnel: w749 -> [w768]
              tunnel: w750 -> [w771] mode=indexing
              tunnel: w751 -> [w770] mode=indexing
              tunnel: [w762] -> w753 mode=indexing
              n344 = call "IMAQ Extract Wavelet Bands"("Image"=w771) -> ("LL"=w773:sgl[][], "HH"=w767:sgl[][])  [unwired: 6 in, 7 out]
              n345 = call "IMAQ Extract Wavelet Bands"("Image"=w770) -> ("LL"=w772:sgl[][], "HH"=w766:sgl[][])  [unwired: 6 in, 7 out]
              n346 = Add(x=w773, y=w772) -> (x+y=w765:sgl[][])
              n347 = Add(x=w767, y=w766) -> (x+y=w764:sgl[][])
              n348 = Add(x=w765, y=w764) -> (x+y=w763:sgl[][])
              n349 = Divide(x=w763, y=w768) -> (x/y=w769:dbl[][])
              n350 = call "IMAQ ArrayToImage"("Image Pixels (U8)"=w769, "Image"=w774) -> ("Image Out"=w762:T2)  [unwired: 8 in, 1 out]
            }
            n351 = Index Array(array=w733, index=10) -> (element=w731:T2)
            n352 = call "IMAQ GetImageInfo"("Image"=w740) -> ("Y Resolution"=w738:i32, "X Resolution"=w739:i32)  [unwired: 3 in, 6 out]
            n353 = call "IMAQ SetImageSize"("Y Resolution"=w738, "X Resolution"=w739, "Image"=w731) -> ("Image Out"=w744:T2)  [unwired: 2 in, 1 out]
            n354 = Index Array(array=w753) -> (element #1=w743:T2, element #2=w742:T2, element #3=w741:T2)  [unwired: 3 in]
            n355 = call "IMAQ ReplaceColorPlane"("Image Src"=w744, "Color Mode"=w737, "Red or Hue Plane"=w743, "Green or Sat Plane"=w742, "Blue or Luma or Val or Inten Plane"=w741) -> ("Image Dst Out"=w732:T2)  [unwired: 9 in, 1 out]
          }
        }
        "Blended ROI" <- w389
      }
      frame #9 {
        # "Measuring the elapsed time for the blending process."
        n356 = local read "Flat Fielding End Time"() -> (w776:dbl)
        n357 = Get Date/Time In Seconds() -> (seconds since 1Jan1904=w778:timestamp)
        n358 = To Double Precision Float(number=w778) -> (double precision float=w777:dbl)
        "Blending End Time" <- w777
        n359 = Subtract(x=w777, y=w776) -> (x-y=→"ROI Blending":dbl)
      }
      frame #10 {
        w789 = 0 ("element")
        # "Panorama Generation:\n\nCreating the panorama destination.\nSetting the size based on the entire images' sizes.\nPositioning the left and right images.\nPositioning the blended ROI.\nProjecting the images onto the panorama destination."
        n360 = local read "Blended ROI"() -> (w783:T2)
        n361 = local read "Wrapped X"() -> (w780:i32)
        n362 = local read "Wrapping Factor"() -> (w794:i32)
        n363 = local read "ROI_X"() -> (w782:i32)
        n364 = Multiply(x=w780, y=2) -> (x*y=w804:i32)
        n365 = Index Array(array=w786, index=11) -> (element=w805:T2)
        n366 = local read "Left corrected, adjusted, and wrapped image"() -> (w800:T2)
        n367 = local read "Wrapped Y"() -> (w781:i32)
        n368 = Subtract(x=w780, y=w782) -> (x-y=w798:i32)
        n369 = Subtract(x=w804, y=w782) -> (x-y=w792:i32)
        n370 = Less Or Equal?(x=w794, y=7) -> (x <= y?=w795:bool)
        n371 = local read "Right corrected, adjusted, and wrapped image"() -> (w799:T2)
        n372 = case shown="False" w795 {
          tunnel: w792 -> [w809 w822]
          tunnel: w794 -> [w808 w820]
          tunnel: [w807 w821] -> w779
          tunnel: w781 -> [w806 w818]
          frame True {
            n373 = Subtract(x=7, y=w808) -> (x-y=w814:i32)
            n374 = Multiply(x=w814, y=7) -> (x*y=w815:i32)
            n375 = Add(x=20 ("y"), y=w815) -> (x+y=w816:i32)
            n376 = Subtract(x=w806, y=w816) -> (x-y=w817:i32)
            n377 = Build Array(0.0 ("element"), w816, w809, w817) -> (w807:dbl[])
          }
          frame False {
            n378 = Subtract(x=w820, y=8) -> (x-y=w826:i32)
            n379 = Multiply(x=w826, y=5) -> (x*y=w827:i32)
            n380 = Subtract(x=32 ("y"), y=w827) -> (x-y=w828:i32)
            n381 = Subtract(x=w818, y=w828) -> (x-y=w829:i32)
            n382 = Build Array(0.0 ("element"), w828, w822, w829) -> (w821:dbl[])
          }
        }
        n383 = call "IMAQ SetImageSize"("Y Resolution"=w781, "X Resolution"=w792, "Image"=w805) -> ("Image Out"=w803:T2)  [unwired: 2 in, 1 out]
        n384 = Build Array(0.0 ("element"), w789) -> (w796:dbl[])
        n385 = call "IMAQ ImageToImage 2"("Offset Left/Top"=w796, "Image Src (Small)"=w800, "Image Src (Large)"=w803) -> ("Image Dst Out"=w802:T2)  [unwired: 7 in, 1 out]
        n386 = Build Array(w798, w789) -> (w797:i32[])
        n387 = call "IMAQ ImageToImage 2"("Offset Left/Top"=w797, "Image Src (Small)"=w799, "Image Src (Large)"=w802) -> ("Image Dst Out"=w801:T2)  [unwired: 7 in, 1 out]
        n388 = call "IMAQ ImageToImage 2"("Offset Left/Top"=w797, "Image Src (Small)"=w783, "Image Src (Large)"=w801) -> ("Image Dst Out"=w793:T2)  [unwired: 7 in, 1 out]
        n389 = call "IMAQ Extract 2"("Optional Rectangle"=w779, "Image Src"=w793) -> ("error out"=w784:errorcluster, "Image Dst Out"=w785:T2)  [unwired: 8 in]
        "Panorama Image" <- w785
      }
      frame #11 {
        # "Calculating the Frames Per Second (FPS) for the processed output."
        n390 = local read "Start Time"() -> (w833:dbl)
        n391 = Get Date/Time In Seconds() -> (seconds since 1Jan1904=w835:timestamp)
        n392 = To Double Precision Float(number=w835) -> (double precision float=w834:dbl)
        n393 = Subtract(x=w834, y=w833) -> (x-y=w831:dbl)
        n394 = Divide(x=1.0, y=w831) -> (x/y=→"Processed FPS":dbl)
      }
    }
  }
  n395 = call "IMAQ Dispose"("Image"=w16, "error in (no error)"=w15) -> ("error out"=→"error out":errorcluster)  [unwired: 4 in]
